vi "Main1.vi"(11 "Stage control":T2={"Up"=FALSE, "Left"=FALSE, "Right"=FALSE, "Down"=FALSE, "Z Down"=FALSE, "Z Up"=FALSE, "X Step Size(um)"=503.04, "Z step size (um)"=10.0, "Y Step Size(um)"=503.04, "Enable x-axis"=TRUE, "Enable y-axis"=TRUE, "Enable z-axis"=TRUE, "Same step size"=FALSE, "Global step size (um)"=10.0, "stop"=FALSE, "Destination"={"X Position"=-2.48414, "Y Position"=-11.8106, "Z Position"=5.53412}, "Move to destination"=FALSE}) -> (10 "Stage position":T1={"X Position"=-42.4711328125, "Y Position"=0.013554687499999999, "Z Position"=0.03555999999999933})   [LabVIEW 2020]
uses:
  typedefs/typedef_stage_control.ctl
  typedefs/typedef_stage_position.ctl
  typedefs/Laser_toggles__manual_typedef.ctl
  typedefs/typedef_voice_coil_function_generation.ctl
  typedefs/typedef_sawtooth_control.ctl
  typedefs/typedef_acquisition.ctl
  typedefs/typedef_laser_order_control.ctl
  <vilib>/DAQmx/write.llb/DAQmx Write (Analog DBL 1Chan 1Samp).vi
  Global stop DAQ.vi
  Global stop.vi
  Global Z-stack acquistion finished flag.vi
  Global DAQ started.vi
  Global destination achieved.vi
  Global stage boundaries.vi
  <vilib>/DAQmx/create/channels.llb/DAQmx Create Channel (AO-Voltage-Basic).vi
  <vilib>/DAQmx/miscellaneous.llb/DAQmx Fill In Error Info.vi
  Global Counter count.vi
panel:
  in  "error in":errorcluster
  in  "Tab Control":enum32{"Manual setup", "Acquisition", "Debug"}(tab)
  in  "Move Home":bool
  out "FirmwareVersion":string="3.03\r"
  out "Connected":bool
  in  "Laser Toggles":T3 {"Laser 642 nm power" min=0.0 max=5.0 scale=0.0..100.0; "Laser 595 nm power" min=0.0 max=5.0 scale=0.0..100.0; "Laser 560 nm power" min=0.0 max=5.0 scale=0.0..100.0; "Laser 488 nm power" min=0.0 max=5.0 scale=0.0..100.0}
  in  "Voice coil voltage slider":dbl(slide) min=-0.6 max=0.6 scale=-0.6..0.6
  in  "Voice coil \ncontrol mode":T4(ring)
  in  "Voice coil voltage output [V]":dbl min=-0.6 max=0.6 format="%#_3g"
  in  "Voice coil function generation":T5={"File to read"=path "C:/Users/Hannah/Downloads/calibration_0624_25msflyback.txt", "Image acquisition time (ms)"=1000.0, "Flyback time (ms)"=25.0}
  in  "Sawtooth generator":T6={"Amplitude [V]"=0.257, "Offset [V]"=-0.031, "Frequency (Hz)"=1.0} {"Frequency (Hz)" min=-50.0 max=50.0 step=0.00010000000000000003 format="%#_13g"; "Offset [V]" format="%.2p"; "Amplitude [V]" min=-0.7 max=0.7 format="%.2p"}
  in  "Calibrate home":bool
  in  "Abort acquisition":bool
  in  "Acquisition":T7={"Acquire"=FALSE, "Step size X and Y (um)"=598.88, "Number of tiles in X"=1.0, "Number of tiles in Y"=1.0, "Number of slices in Z"=1.0, "Step size Z (um)"=0.2, "Image acquisition time (ms)"=1000.0, "Flyback time (ms)"=25.0, "Moving time between tiles (ms)"=5000.0, "Total progress"=0, "Percentage overlap"=5.0, "Voice coil calibration file"=path "C:/Users/Hannah/Downloads/calibration1_fps_10000_samples_25ms_flyback", "Saved file location"=path "C:/Users/Hannah/Downloads/PositionLog7", "typedef_laser_order_control"={"Laser 560 nm order selection"=0, "Laser 595 nm order selection"=0, "Laser 642 nm order selection"=0, "Laser 488 nm order selection"=1, "Color Box"=60927, "Color Box 2"=12844800, "Color Box 3"=14132992, "Color Box 4"=16715008}, "Z-stack progress"=0} {"Z-stack progress" scale=0.0..100.0; "typedef_laser_order_control"."Laser 488 nm order selection" items=["Not active", "1", "2", "3", "4"]; "typedef_laser_order_control"."Laser 642 nm order selection" items=["Not active", "1", "2", "3", "4"]; "typedef_laser_order_control"."Laser 595 nm order selection" items=["Not active", "1", "2", "3", "4"]; "typedef_laser_order_control"."Laser 560 nm order selection" items=["Not active", "1", "2", "3", "4"]; "Percentage overlap" min=0.1 max=100.0; "Total progress" scale=0.0..100.0}
  out "Error out":errorcluster
  in  "DAQ Setup":enum16{"Test setup", "Microscope"}(ring)=enum."Microscope"
  in  "stop":bool
  out "Number of commands":i32=159
  out "waiting time (ms)":dbl
  out "output cluster":T9={"element"="acquire Zstack", "reference OUT"=refnum, "error OUT"={"status"=FALSE, "code"=0, "source"=""}}
  in  "additional delay":dbl=-97.0
  out "string array":string[](array[string])=["acquireXY", "WAIT2040", "MOVEX+1", "WAIT5000", "acquireXY", "WAIT2040", "MOVEX+1", "WAIT5000", "acquireXY", "WAIT2040", "MOVEX+1", "WAIT5000", "acquireXY", "WAIT2040", "MOVEY-1", "WAIT5000", "acquireXY", "WAIT2040", "MOVEX-1", "WAIT5000", "acquireXY", "WAIT2040", "MOVEX-1", "WAIT5000", "acquireXY", "WAIT2040", "MOVEX-1", "WAIT5000", "acquireXY", "WAIT2040", "MOVEY-1", "WAIT5000", "acquireXY", "WAIT2040", "MOVEX+1", "WAIT5000", "acquireXY", "WAIT2040", "MOVEX+1", "WAIT5000", "acquireXY", "WAIT2040", "MOVEX+1", "WAIT5000", "acquireXY", "WAIT2040", "MOVEY-1", "WAIT5000", "acquireXY", "WAIT2040", "MOVEX-1", "WAIT5000", "acquireXY", "WAIT2040", "MOVEX-1", "WAIT5000", "acquireXY", "WAIT2040", "MOVEX-1", "WAIT5000", "acquireXY", "WAIT2040", "MOVEY-1", "WAIT5000", "acquireXY", "WAIT2040", "MOVEX+1", "WAIT5000", "acquireXY", "WAIT2040", "MOVEX+1", "WAIT5000", "acquireXY", "WAIT2040", "MOVEX+1", "WAIT5000", "acquireXY", "WAIT2040", "MOVEY-1", "WAIT5000", "acquireXY", "WAIT2040", "MOVEX-1", "WAIT5000", "acquireXY", "WAIT2040", "MOVEX-1", "WAIT5000", "acquireXY", "WAIT2040", "MOVEX-1", "WAIT5000", "acquireXY", "WAIT2040", "MOVEY-1", "WAIT5000", "acquireXY", "WAIT2040", "MOVEX+1", "WAIT5000", "acquireXY", "WAIT2040", "MOVEX+1", "WAIT5000", "acquireXY", "WAIT2040", "MOVEX+1", "WAIT5000", "acquireXY", "WAIT2040", "MOVEY-1", "WAIT5000", "acquireXY", "WAIT2040", "MOVEX-1", "WAIT5000", "acquireXY", "WAIT2040", "MOVEX-1", "WAIT5000", "acquireXY", "WAIT2040", "MOVEX-1", "WAIT5000", "acquireXY", "WAIT2040", "MOVEY-1", "WAIT5000", "acquireXY", "WAIT2040", "MOVEX+1", "WAIT5000", "acquireXY", "WAIT2040", "MOVEX+1", "WAIT5000", "acquireXY", "WAIT2040", "MOVEX+1", "WAIT5000", "acquireXY", "WAIT2040", "MOVEY-1", "WAIT5000", "acquireXY", "WAIT2040", "MOVEX-1", "WAIT5000", "acquireXY", "WAIT2040", "MOVEX-1", "WAIT5000", "acquireXY", "WAIT2040", "MOVEX-1", "WAIT5000", "acquireXY", "WAIT2040", "end"]
  out "String":string="X+1 movement"
  out "Z-stack start position":T1
  in  "X-direction":enum16{"Up", "Down"}(ring)
  in  "Y-direction":enum16{"Left", "Right"}(ring)=enum."Right"
  out "Numeric 2":i32
  out "Boolean":bool
  out "Numeric 3":i32
  out "Numeric 4":i32
  out "Stage position OUT":T1
  out "Stage position OUT 2":T1
  in  "FOV (um)":dbl=630.4 format="%#_13g"
  out "current position in string array":i32=11
  in  "Camera trigger initial delay [ms]":dbl format="%.6f"
  out "Global Counter count":dbl
  out "Numeric":i32
  in  "SPIIPLUSCOM660Lib.IAsyncChannel":refnum<k7>
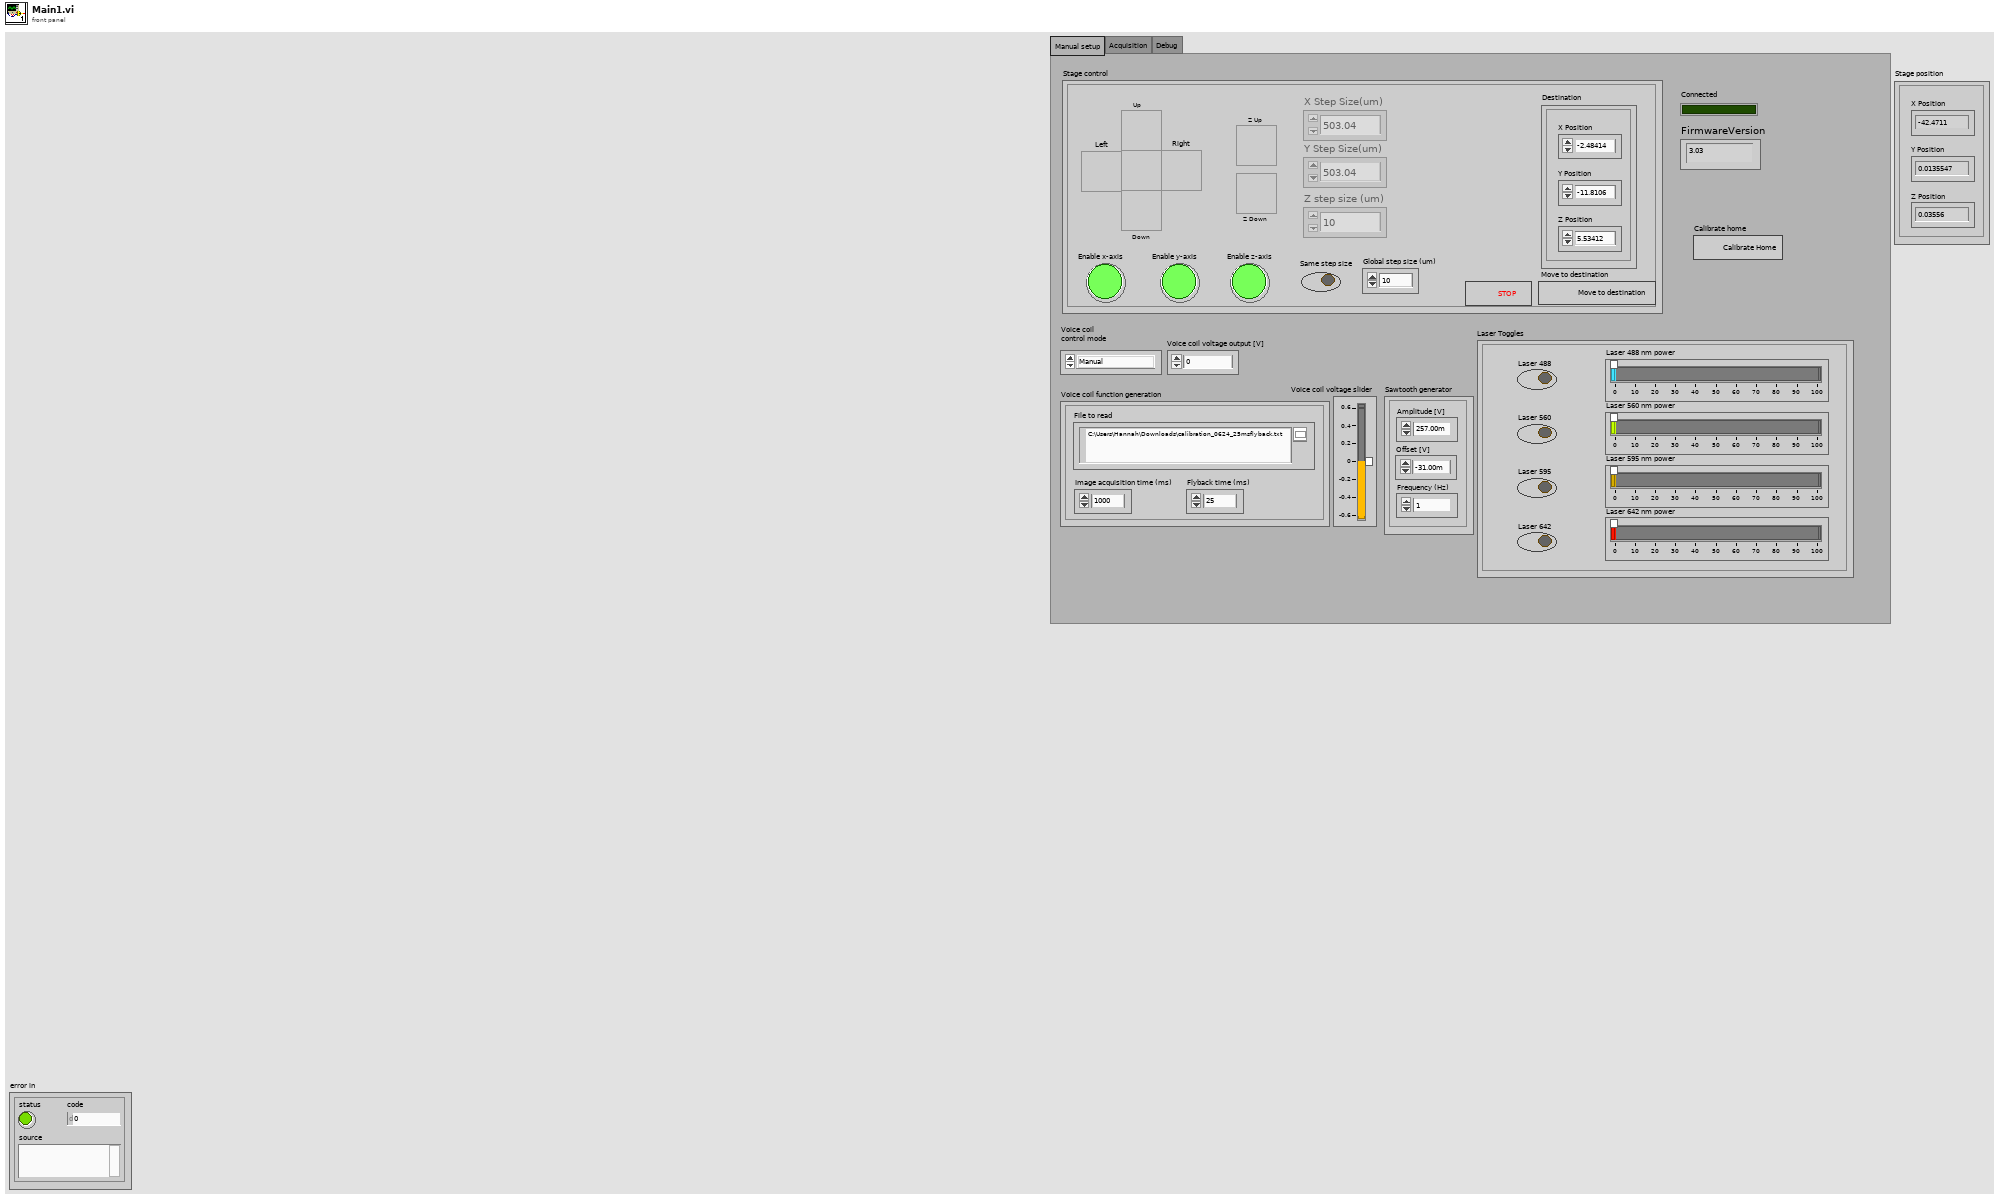
[diagram p1: front panel]
types:
  T1 = typedef "typedef_stage_position.ctl" = cluster{"X Position":dbl, "Y Position":dbl, "Z Position":dbl}
  T2 = typedef "typedef_stage_control.ctl" = cluster{"Up":bool, "Left":bool, "Right":bool, "Down":bool, "Z Down":bool, "Z Up":bool, "X Step Size(um)":dbl, "Z step size (um)":dbl, "Y Step Size(um)":dbl, "Enable x-axis":bool, "Enable y-axis":bool, "Enable z-axis":bool, "Same step size":bool, "Global step size (um)":dbl, "stop":bool, "Destination":T1, "Move to destination":bool}
  T3 = typedef "Laser_toggles__manual_typedef.ctl" = cluster{"Laser 488 nm power":dbl, "Laser 560 nm power":dbl, "Laser 595 nm power":dbl, "Laser 642 nm power":dbl, "Laser 560 ":bool, "Laser 595 ":bool, "Laser 642 ":bool, "Laser 488 ":bool}
  T4 = enum16{"Manual", "Saw tooth function", "From file"}
  T5 = typedef "typedef_voice_coil_function_generation.ctl" = cluster{"File to read":path, "Image acquisition time (ms)":dbl, "Flyback time (ms)":dbl}
  T6 = typedef "typedef_sawtooth_control.ctl" = cluster{"Amplitude [V]":dbl, "Offset [V]":dbl, "Frequency (Hz)":dbl}
  T7 = typedef "typedef_acquisition.ctl" = cluster{"Acquire":bool, "Step size X and Y (um)":dbl, "Number of tiles in X":dbl, "Number of tiles in Y":dbl, "Number of slices in Z":dbl, "Step size Z (um)":dbl, "Image acquisition time (ms)":dbl, "Flyback time (ms)":dbl, "Moving time between tiles (ms)":dbl, "Total progress":u8, "Percentage overlap":dbl, "Voice coil calibration file":path, "Saved file location":path, "typedef_laser_order_control":T8, "Z-stack progress":u8}
  T8 = typedef "typedef_laser_order_control.ctl" = cluster{"Laser 560 nm order selection":u16, "Laser 595 nm order selection":u16, "Laser 642 nm order selection":u16, "Laser 488 nm order selection":u16, "Color Box":u32, "Color Box 2":u32, "Color Box 3":u32, "Color Box 4":u32}
  T9 = cluster{"element":string, "reference OUT":refnum<k7>, "error OUT":errorcluster}
  T10 = enum16{"Initialize", "Verify connection", "Running", "Closing"}
  T11 = enum16{"Turn off X and Y", "Manually move stage 1", "Manually move stage 2", "Enable Home button", "Activate X and Y"}
  T12 = enum8{"Enabled", "Disabled", "Disabled and Grayed Out"}
  T13 = typedef "typedef_boundaries.ctl" = cluster{"X lower bound":dbl, "X upper bound":dbl, "Y lower bound":dbl, "Y upper bound ":dbl, "Z lower bound":dbl, "Z upper bound ":dbl}
  T14 = typedef "DAQ_channel_typedef.ctl" = cluster{"CO.Pulse.Term":tag, "Voice coil analog output":tag, "counter":tag, "CO.Pulse.Term 2":tag, "AOTF lines":tag, "counter 2":tag, "CO.Pulse.Term 3":tag, "counter 3":tag}
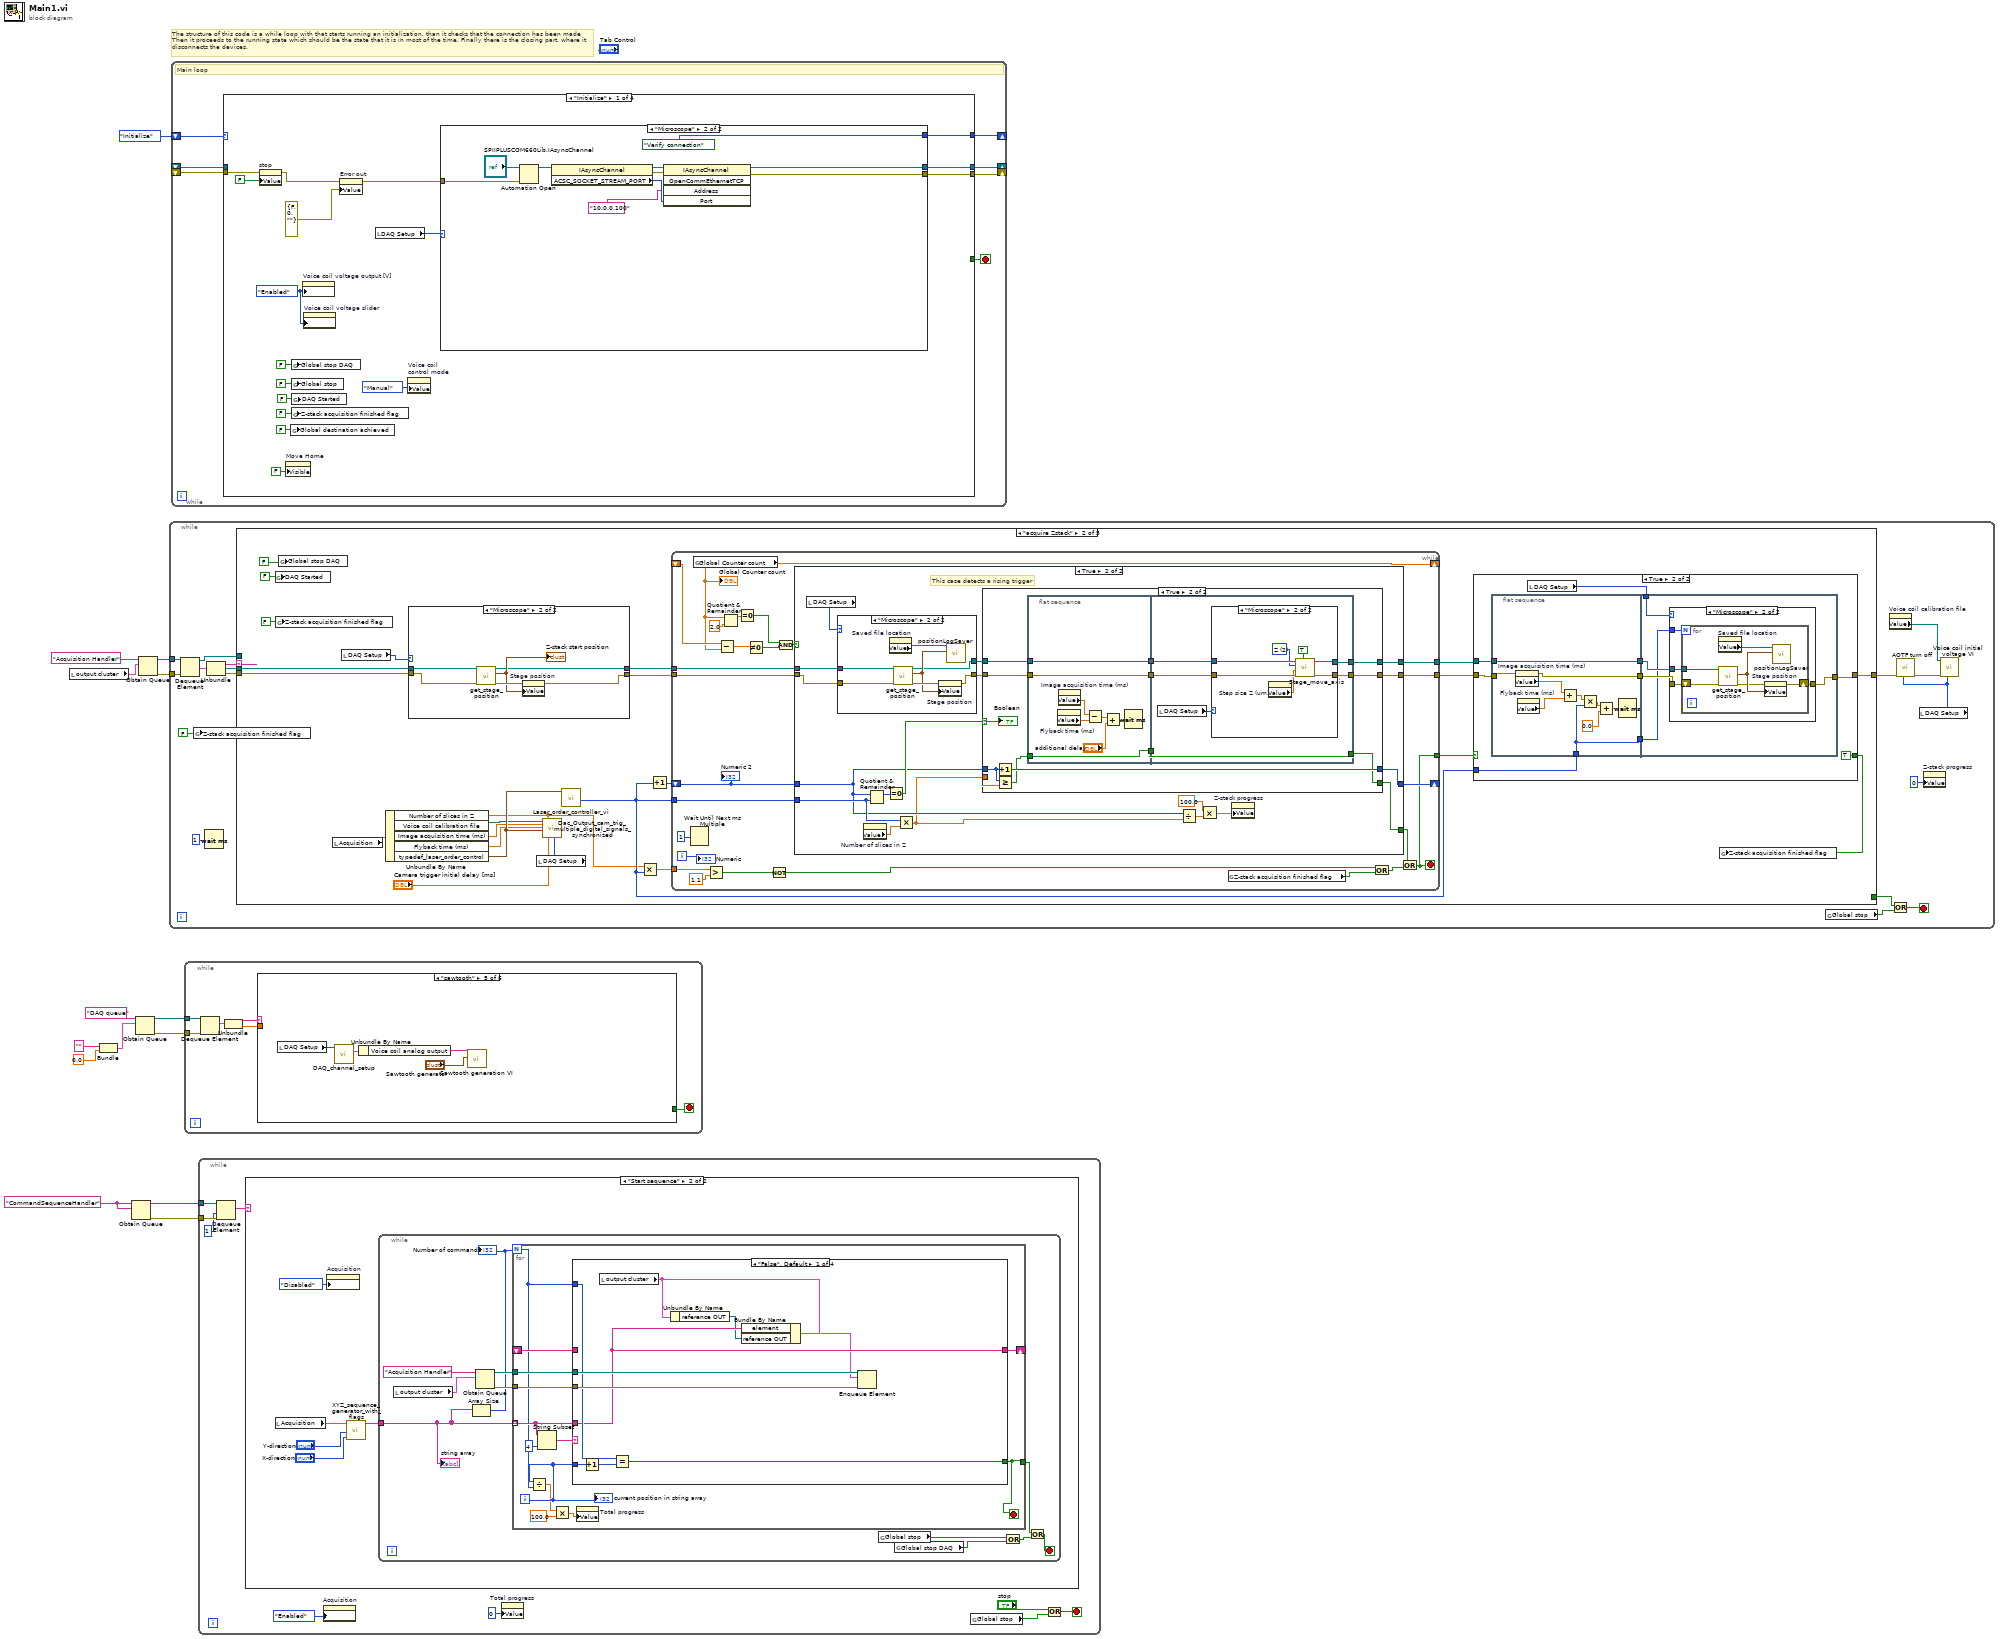
[diagram p0: block diagram]
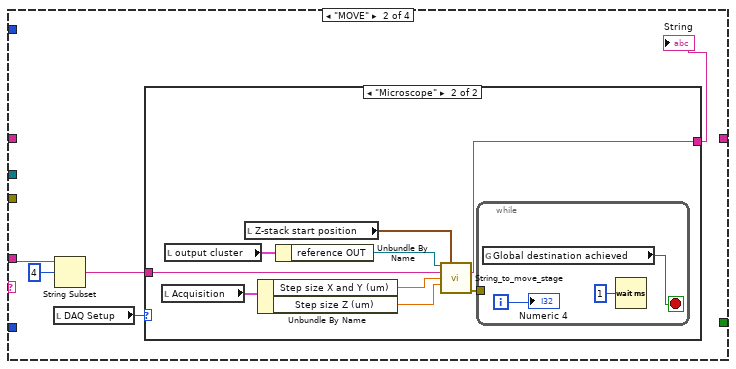
[diagram p3: hidden frame]
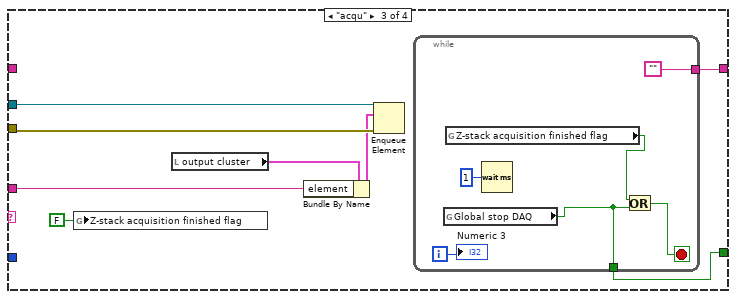
[diagram p5: hidden frame]
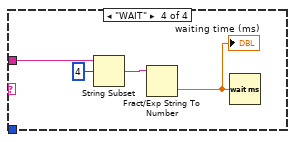
[diagram p6: hidden frame]
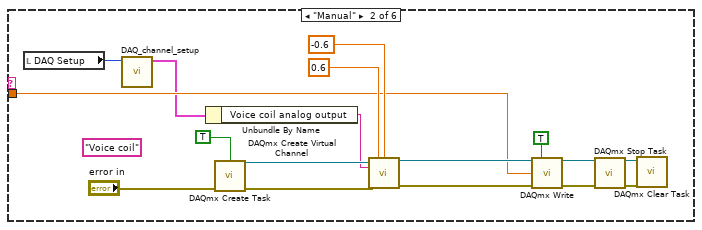
[diagram p8: hidden frame]
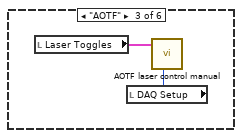
[diagram p9: hidden frame]
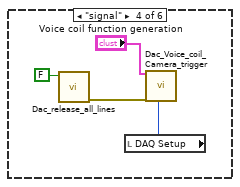
[diagram p10: hidden frame]
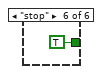
[diagram p11: hidden frame]
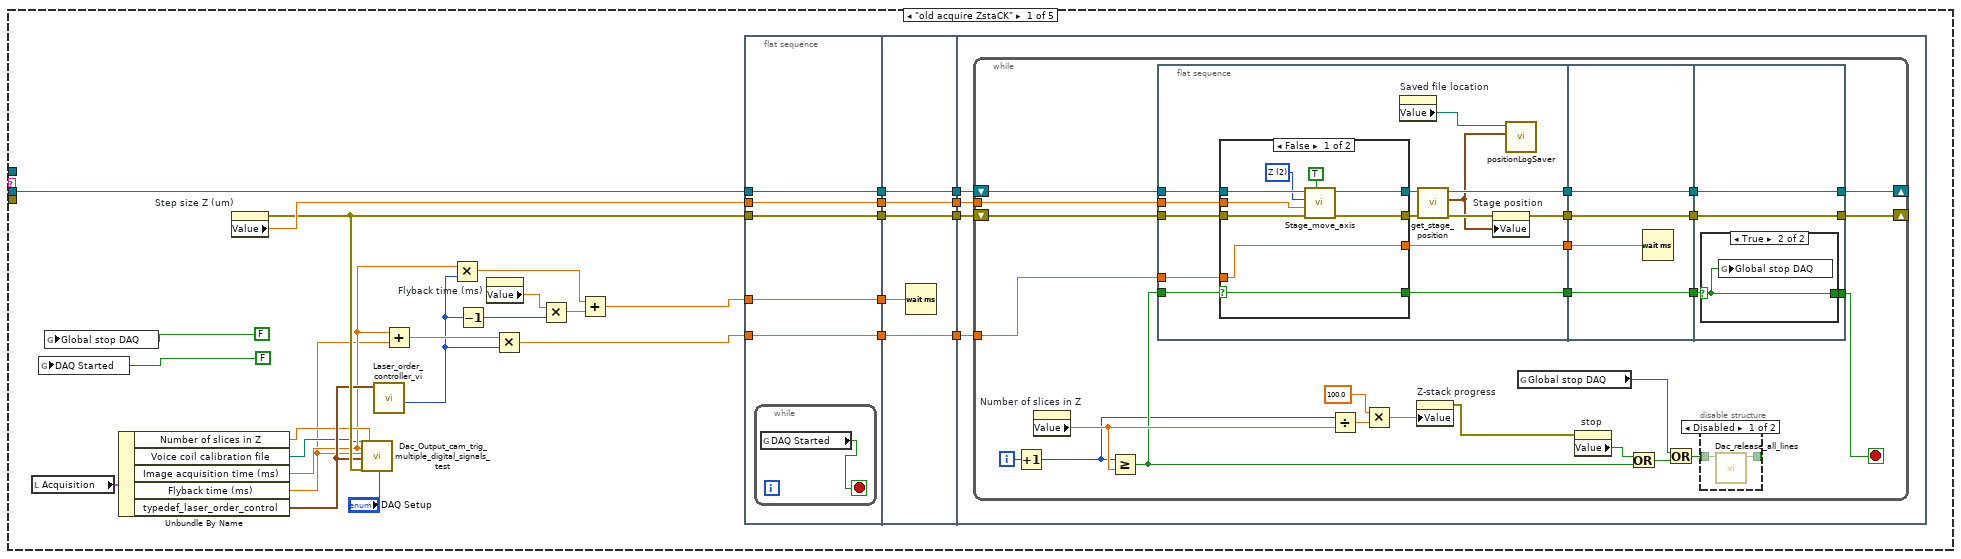
[diagram p12: hidden frame]
diagram:
  w2 = "CommandSequenceHandler" ("name (unnamed)")
  # "The structure of this code is a while loop with that starts running an initialization, than it checks that the connection has been made\nThen it proceeds to the running state which should be the state that it is in most of the time. Finally there is the closing part, where it\ndisconnects the devices."
  n1 = local read "output cluster"() -> (w1:T9)
  n2 = Bundle("", 0.0) -> (w10:cluster{string, dbl})  [unwired: 1 in]
  n3 = Obtain Queue(name (unnamed)=w2, element data type=w2) -> (queue out=w4:refnum<queue>, error out=w3:errorcluster)  [unwired: 3 in, 1 out]
  n4 = Obtain Queue(name (unnamed)="DAQ queue", element data type=w10) -> (queue out=w8:refnum<queue>, error out=w7:errorcluster)  [unwired: 3 in, 1 out]
  n5 = Obtain Queue(name (unnamed)="Acquisition Handler", element data type=w1) -> (queue out=w12:refnum<queue>, error out=w11:errorcluster)  [unwired: 3 in, 1 out]
  n6 = while {
    tunnel: w12 -> [w31]
    tunnel: w11 -> [w30]
    stop <- w19 stop-if-true
    n7 = Dequeue Element(queue=w31, error in (no error)=w30) -> (queue out=w25:refnum<queue>, element=w29:T9)  [unwired: 1 in, 2 out]
    n8 = global write "Global Z-stack acquistion finished flag.vi" "Z-stack acquisition finished flag"(FALSE ("Z-stack acquisition finished flag")) -> ()
    n9 = Wait (ms)(milliseconds to wait=u32 1) -> ()  [unwired: 1 out]
    n10 = Unbundle(w29) -> ("element"=w28:string, "reference OUT"=w27:refnum<k7>, "error OUT"=w26:errorcluster)
    n11 = case shown="\"acquire Zstack\"" w28 {
      tunnel: w27 -> [w60 w162 _ _ _]
      tunnel: w26 -> [_ w161 _ _ _]
      tunnel: [_ _ _ _ TRUE] -> w18
      tunnel: w25 -> [_ _ _ _ _]
      tunnel: [_ w152 _ _ _] -> w15
      frame "old acquire ZstaCK" {
        n12 = local read "Acquisition"() -> (w36:T7)
        n13 = global write "Global DAQ started.vi" "DAQ Started"(FALSE ("DAQ Started")) -> ()
        n14 = global write "Global stop DAQ.vi" "Global stop DAQ"(FALSE ("Global stop DAQ")) -> ()
        n15 = Unbundle By Name(w36) -> ("Number of slices in Z"=w35:dbl, "Voice coil calibration file"=w33:path, "Image acquisition time (ms)"=w34:dbl, "Flyback time (ms)"=w32:dbl, "typedef_laser_order_control"=w37:T8)
        n16 = property on="Step size Z (um)" class="DigNum (strict)"() -> (error out=w58:errorcluster, "Value"=w59:dbl)  [unwired: 2 in, 1 out]
        n17 = call "Dac_Output_cam_trig_multiple_digital_signals_test.vi"("File to read"=w33, "Image acquisition time (ms)"=w34, "Delay between frames"=w32, "typedef_laser_order_control"=w37, "error in"=w58, "Number of slices"=w35, "Setup"="DAQ Setup") -> ()  [unwired: 12 in, 1 out]
        n18 = call "Laser_order_controller_vi.vi"("typedef_laser_order_control"=w37) -> ("Active lasers"=w39:i16)  [unwired: 8 in, 2 out]
        n19 = Add(x=w34, y=w32) -> (x+y=w57:dbl)
        n20 = Multiply(x=w34, y=w39) -> (x*y=w38:dbl)
        n21 = Decrement(x=w39) -> (x-1=w54:i16)
        n22 = property on="Flyback time (ms)" class="DigNum (strict)"() -> ("Value"=w53:dbl)  [unwired: 2 in, 2 out]
        n23 = Multiply(x=w57, y=w39) -> (x*y=w51:dbl)
        n24 = Multiply(x=w53, y=w54) -> (x*y=w52:dbl)
        n25 = Add(x=w38, y=w52) -> (x+y=w46:dbl)
        n26 = flat-sequence {
          tunnel: w46 -> [w61]
          tunnel: w51 -> [w62]
          tunnel: w58 -> [w63]
          tunnel: w59 -> [w64]
          tunnel: w60 -> [w65]
          tunnel: [w65] -> w45
          tunnel: [w64] -> w44
          tunnel: [w63] -> w43
          tunnel: [w62] -> w42
          tunnel: [w61] -> w41
          tunnel: [w71] -> w50
          tunnel: [w70] -> w49
          tunnel: [w69] -> w48
          tunnel: [w68] -> w47
          tunnel: w45 -> [w71]
          tunnel: w44 -> [w70]
          tunnel: w43 -> [w69]
          tunnel: w42 -> [w68]
          tunnel: w41 -> [w67]
          tunnel: w50 -> [w75]
          tunnel: w49 -> [w74]
          tunnel: w48 -> [w73]
          tunnel: w47 -> [w72]
          frame #0 {
            n27 = while {
              stop <- w66 stop-if-true
              n28 = global read "Global DAQ started.vi" "DAQ Started"() -> (w66:bool)
            }
          }
          frame #1 {
            n29 = Wait (ms)(milliseconds to wait=w67) -> ()  [unwired: 1 out]
          }
          frame #2 {
            n30 = while {
              shift-right: [w100] -> _
              shift-left: w75 -> [w101]
              shift-right: [w84] -> _
              shift-left: w73 -> [w90]
              tunnel: w74 -> [w96]
              tunnel: w72 -> [w88]
              i -> [w82]
              stop <- w77 stop-if-true
              n31 = Increment(x=w82) -> (x+1=w76:i32)
              n32 = property on="Number of slices in Z" class="DigNum (strict)"() -> ("Value"=w94:dbl)  [unwired: 2 in, 2 out]
              n33 = Greater Or Equal?(x=w76, y=w94) -> (x >= y?=w83:bool)
              n34 = flat-sequence {
                tunnel: w101 -> [w118]
                tunnel: w96 -> [w115]
                tunnel: [w117] -> w93
                tunnel: [w116] -> w92
                tunnel: w90 -> [w111]
                tunnel: w83 -> [w110]
                tunnel: w88 -> [w109]
                tunnel: [w108] -> w89
                tunnel: [w106] -> w78
                tunnel: w93 -> [w135]
                tunnel: w92 -> [w134]
                tunnel: w89 -> [w132]
                tunnel: [w135] -> w81
                tunnel: [w134] -> w80
                tunnel: [w133] -> w79
                tunnel: w78 -> [w133]
                tunnel: [w138] -> w84
                tunnel: [w139] -> w100
                tunnel: w81 -> [w139]
                tunnel: w80 -> [w138]
                tunnel: w79 -> [w137]
                tunnel: [w136] -> w77
                frame #0 {
                  n35 = case shown="False" w110 {
                    selector: w110 -> [w120 w129]
                    tunnel: w118 -> [w127 w131]
                    tunnel: w115 -> [w126 _]
                    tunnel: [w123 w131] -> w114
                    tunnel: [w122 w130] -> w113
                    tunnel: w111 -> [w121 w130]
                    tunnel: w109 -> [w119 w128]
                    tunnel: [w119 w128] -> w108
                    tunnel: [w120 w129] -> w106
                    frame False {
                      w125 = u16 2 items=["X", "Y", "Z"] ("Axes Select")
                      n36 = call "Stage_move_axis.vi"("Direction true means positive increment"=TRUE, "error in (no error)"=w121, "Distance micrometer"=w126, "Axes Select"=w125, "reference IN"=w127) -> ("error OUT"=w122:errorcluster, "reference OUT"=w123:refnum<k7>)  [unwired: 5 in]
                    }
                    frame True {
                      # "Last acquisition should not wait"
                    }
                  }
                  n37 = property on="Saved file location" class="Path"() -> ("Value"=w105:path)  [unwired: 2 in, 2 out]
                  n38 = call "get_stage_position.vi"("error IN"=w113, "reference IN"=w114) -> ("error OUT"=w112:errorcluster, "Stage position OUT"=w107:T1, "reference OUT"=w117:refnum<k7>)  [unwired: 7 in]
                  n39 = property on="Stage position" class="Clust (strict)"(error in=w112, "Value"=w107) -> (error out=w116:errorcluster)  [unwired: 1 in, 1 out]
                  n40 = call "positionLogSaver.vi"("Stage position"=w107, "file path (use dialog)"=w105) -> ()  [unwired: 10 in]
                }
                frame #1 {
                  n41 = Wait (ms)(milliseconds to wait=w132) -> ()  [unwired: 1 out]
                }
                frame #2 {
                  n42 = case shown="True" w137 {
                    selector: w137 -> [w140 w141]
                    tunnel: [w140 w141] -> w136
                    frame False {
                    }
                    frame True {
                      n43 = global write "Global stop DAQ.vi" "Global stop DAQ"(w141) -> ()
                    }
                  }
                }
              }
              n44 = Divide(x=w76, y=w94) -> (x/y=w98:dbl)
              n45 = Multiply(x=100.0 ("y"), y=w98) -> (x*y=w95:dbl)
              n46 = property on="Z-stack progress" class="Slide (strict)"("Value"=w95) -> (error out=w91:errorcluster)  [unwired: 2 in, 1 out]
              n47 = global read "Global stop DAQ.vi" "Global stop DAQ"() -> (w86:bool)
              n48 = property on="stop" class="Bool (strict)"(error in=w91) -> ("Value"=w99:bool)  [unwired: 1 in, 2 out]
              n49 = Or(x=w99, y=w83) -> (x .or. y?=w87:bool)
              n50 = Or(x=w86, y=w87) -> (x .or. y?=w85:bool)
              n51 = disable-structure shown="Disabled" {
                disable-tunnel: w85 -> [w103 w104]
                disable-tunnel: [w102 w104] -> _
                frame Disabled {
                  n52 = call "Dac_release_all_lines.vi"("Release all DAQ lines"=w103) -> ("Finished"=w102:bool)  [unwired: 9 in, 1 out]
                }
                frame Enabled {
                }
              }
            }
          }
        }
      }
      frame "acquire Zstack" {
        n53 = global write "Global DAQ started.vi" "DAQ Started"(FALSE ("DAQ Started")) -> ()
        n54 = global write "Global Z-stack acquistion finished flag.vi" "Z-stack acquisition finished flag"(FALSE ("Z-stack acquisition finished flag")) -> ()
        n55 = global write "Global stop DAQ.vi" "Global stop DAQ"(FALSE ("Global stop DAQ")) -> ()
        n56 = local read "Acquisition"() -> (w148:T7)
        n57 = local read "DAQ Setup"() -> (w157:enum16{"Test setup", "Microscope"})
        n58 = Unbundle By Name(w148) -> ("Number of slices in Z"=w143:dbl, "Voice coil calibration file"=w146:path, "Image acquisition time (ms)"=w144:dbl, "Flyback time (ms)"=w145:dbl, "typedef_laser_order_control"=w147:T8)
        n59 = case shown="\"Microscope\"" w157 {
          tunnel: w162 -> [w204 w208]
          tunnel: w161 -> [w203 w207]
          tunnel: [w203 w206] -> w160
          tunnel: [w204 w205] -> w159
          frame "Test setup", Default {
          }
          frame "Microscope" {
            n60 = call "get_stage_position.vi"("error IN"=w207, "reference IN"=w208) -> ("error OUT"=w210:errorcluster, "Stage position OUT"=w209:T1, "reference OUT"=w205:refnum<k7>)  [unwired: 7 in]
            "Z-stack start position" <- w209
            n61 = property on="Stage position" class="Clust (strict)"(error in=w210, "Value"=w209) -> (error out=w206:errorcluster)  [unwired: 1 in, 1 out]
          }
        }
        n62 = local read "DAQ Setup"() -> (w163:enum16{"Test setup", "Microscope"})
        n63 = call "Dac_Output_cam_trig_multiple_digital_signals_synchronized.vi"("File to read"=w146, "Image acquisition time (ms)"=w144, "Delay between frames (ms)"=w145, "typedef_laser_order_control"=w147, "Number of slices"=w143, "Camera trigger initial delay [ms]"="Camera trigger initial delay [ms]", "Setup"=w163) -> ()  [unwired: 12 in, 1 out]
        n64 = call "Laser_order_controller_vi.vi"("typedef_laser_order_control"=w147) -> ("Active lasers"=w149:i16)  [unwired: 8 in, 2 out]
        n65 = Multiply(x=w143, y=w149) -> (x*y=w155:dbl)
        n66 = Increment(x=w149) -> (x+1=w150:i16)
        n67 = while {
          shift-right: [w226] -> _
          shift-left: _ -> [w228]
          tunnel: w159 -> [w234]
          tunnel: w160 -> [w233]
          shift-right: [w229] -> _
          shift-left: w150 -> [w230]
          tunnel: w149 -> [w224]
          tunnel: [w223] -> w154
          tunnel: w155 -> [w222]
          tunnel: [w215] -> w156
          tunnel: [w214] -> w153
          i -> [w231]
          stop <- w215 stop-if-true
          n68 = Wait Until Next ms Multiple(millisecond multiple=u32 1) -> ()  [unwired: 1 out]
          n69 = global read "Global Counter count.vi" "Global Counter count"() -> (w226:dbl)
          "Global Counter count" <- w226
          n70 = Greater?(x=w222, y=1.1) -> (0:w217:bool)
          n71 = Subtract(x=w228, y=w226) -> (x-y=w235:dbl)
          n72 = Quotient & Remainder(x=w226, y=2.0) -> (x-y*floor(x/y)=w225:dbl)  [unwired: 1 out]
          n73 = Equal To 0?(x=w225) -> (x = 0?=w219:bool)
          n74 = Not Equal To 0?(x=w235) -> (x != 0?=w218:bool)
          n75 = Not(x=w217) -> (.not. x?=w212:bool)
          n76 = And(x=w219, y=w218) -> (x .and. y?=w220:bool)
          n77 = case shown="True" w220 {
            tunnel: w234 -> [w236 w242]
            tunnel: w233 -> [w237 w243]
            tunnel: w230 -> [w238 w247]
            tunnel: [w238 w246] -> w229
            tunnel: w224 -> [_ w250]
            tunnel: [_ w244] -> w216
            tunnel: [w237 w249] -> w223
            tunnel: [w236 w248] -> w214
            frame False {
            }
            frame True {
              # "This case detects a rising trigger"
              n78 = local read "DAQ Setup"() -> (w239:enum16{"Test setup", "Microscope"})
              n79 = case shown="\"Microscope\"" w239 {
                tunnel: w243 -> [w257 w262]
                tunnel: w242 -> [w258 w261]
                tunnel: [w257 w260] -> w241
                tunnel: [w258 w259] -> w240
                frame "Test setup", Default {
                }
                frame "Microscope" {
                  n80 = property on="Saved file location" class="Path"() -> ("Value"=w265:path)  [unwired: 2 in, 2 out]
                  n81 = call "get_stage_position.vi"("error IN"=w262, "reference IN"=w261) -> ("error OUT"=w264:errorcluster, "Stage position OUT"=w263:T1, "reference OUT"=w259:refnum<k7>)  [unwired: 7 in]
                  n82 = property on="Stage position" class="Clust (strict)"(error in=w264, "Value"=w263) -> (error out=w260:errorcluster)  [unwired: 1 in, 1 out]
                  n83 = call "positionLogSaver.vi"("Stage position"=w263, "file path (use dialog)"=w265) -> ()  [unwired: 10 in]
                }
              }
              n84 = property on="Number of slices in Z" class="DigNum (strict)"() -> ("Value"=w251:dbl)  [unwired: 2 in, 2 out]
              n85 = Quotient & Remainder(x=w247, y=w250) -> (x-y*floor(x/y)=w253:i16)  [unwired: 1 out]
              n86 = Equal To 0?(x=w253) -> (x = 0?=w252:bool)
              n87 = Multiply(x=w250, y=w251) -> (x*y=w245:dbl)
              n88 = case shown="True" w252 {
                selector: w252 -> [w270 w281]
                tunnel: [w271 w284] -> w249
                tunnel: w240 -> [w269 w283]
                tunnel: w241 -> [w271 w282]
                tunnel: [w269 w278] -> w248
                tunnel: w247 -> [w267 w276]
                tunnel: [w268 w277] -> w246
                tunnel: w245 -> [_ w275]
                tunnel: [FALSE w272] -> w244
                frame False {
                  n89 = local write "Boolean"(w270) -> ()
                  n90 = Increment(x=w267) -> (x+1=w268:i16)
                }
                frame True {
                  n91 = Increment(x=w276) -> (x+1=w277:i16)
                  n92 = Greater Or Equal?(x=w276, y=w275) -> (x >= y?=w274:bool)
                  n93 = flat-sequence {
                    tunnel: w282 -> [w291]
                    tunnel: w283 -> [w292]
                    tunnel: [w292] -> w280
                    tunnel: [w291] -> w279
                    tunnel: w274 -> [w285]
                    tunnel: [w285] -> w273
                    tunnel: [w298] -> w284
                    tunnel: w280 -> [w297]
                    tunnel: w279 -> [w296]
                    tunnel: [w294] -> w278
                    tunnel: [w293] -> w272
                    tunnel: w273 -> [w293]
                    frame #0 {
                      n94 = property on="Flyback time (ms)" class="DigNum (strict)"() -> ("Value"=w289:dbl)  [unwired: 2 in, 2 out]
                      n95 = property on="Image acquisition time (ms)" class="DigNum (strict)"() -> ("Value"=w290:dbl)  [unwired: 2 in, 2 out]
                      n96 = Subtract(x=w290, y=w289) -> (x-y=w287:dbl)
                      n97 = Add(x=w287, y="additional delay") -> (x+y=w288:dbl)
                      n98 = Wait (ms)(milliseconds to wait=w288) -> ()  [unwired: 1 out]
                    }
                    frame #1 {
                      n99 = local read "DAQ Setup"() -> (w295:enum16{"Test setup", "Microscope"})
                      n100 = case shown="\"Microscope\"" w295 {
                        tunnel: [w300 w301] -> w298
                        tunnel: w297 -> [w299 w307]
                        tunnel: w296 -> [w300 w306]
                        tunnel: [w299 w302] -> w294
                        frame "Test setup", Default {
                        }
                        frame "Microscope" {
                          w305 = u16 2 items=["X", "Y", "Z"] ("Axes Select")
                          n101 = property on="Step size Z (um)" class="DigNum (strict)"() -> ("Value"=w303:dbl)  [unwired: 2 in, 2 out]
                          n102 = call "Stage_move_axis.vi"("Direction true means positive increment"=TRUE, "error in (no error)"=w306, "Distance micrometer"=w303, "Axes Select"=w305, "reference IN"=w307) -> ("error OUT"=w301:errorcluster, "reference OUT"=w302:refnum<k7>)  [unwired: 5 in]
                        }
                      }
                    }
                  }
                  "Boolean" <- w281
                }
              }
              n103 = Divide(x=w247, y=w245) -> (x/y=w256:dbl)
              n104 = Multiply(x=100.0 ("y"), y=w256) -> (x*y=w254:dbl)
              n105 = property on="Z-stack progress" class="Slide (strict)"("Value"=w254) -> ()  [unwired: 2 in, 2 out]
            }
          }
          n106 = global read "Global Z-stack acquistion finished flag.vi" "Z-stack acquisition finished flag"() -> (w211:bool)
          n107 = Or(x=w212, y=w211) -> (x .or. y?=w213:bool)
          n108 = Or(x=w216, y=w213) -> (x .or. y?=w215:bool)
          "Numeric" <- w231
          "Numeric 2" <- w230
        }
        n109 = case shown="True" w156 {
          selector: w156 -> [w167 _]
          tunnel: [w167 TRUE] -> w151
          tunnel: w149 -> [_ w172]
          tunnel: w154 -> [w166 w175]
          tunnel: w153 -> [_ w169]
          tunnel: [w166 w171] -> w152
          frame False {
          }
          frame True {
            n110 = flat-sequence {
              tunnel: w175 -> [w184]
              tunnel: w172 -> [w177]
              tunnel: [w183] -> w174
              tunnel: [w178] -> w170
              tunnel: w169 -> [w178]
              tunnel: [w177] -> w168
              tunnel: w174 -> [w190]
              tunnel: w173 -> [w191]
              tunnel: [w189] -> w171
              tunnel: w170 -> [w188]
              tunnel: w168 -> [w187]
              frame #0 {
                n111 = property on="Image acquisition time (ms)" class="DigNum (strict)"(error in=w184) -> (error out=w183:errorcluster, "Value"=w186:dbl)  [unwired: 1 in, 1 out]
                n112 = property on="Flyback time (ms)" class="DigNum (strict)"() -> ("Value"=w180:dbl)  [unwired: 2 in, 2 out]
                n113 = Add(x=w186, y=w180) -> (x+y=w185:dbl)
                n114 = Multiply(x=w185, y=w177) -> (x*y=w182:dbl)
                n115 = Add(x=w182, y=0.0) -> (x+y=w181:dbl)
                n116 = Wait (ms)(milliseconds to wait=w181) -> ()  [unwired: 1 out]
              }
              frame #1 {
                n117 = case shown="\"Microscope\"" w191 {
                  tunnel: [w192 w196] -> w189
                  tunnel: w190 -> [w192 w195]
                  tunnel: w188 -> [_ w194]
                  tunnel: w187 -> [_ w193]
                  frame "Test setup", Default {
                  }
                  frame "Microscope" {
                    n118 = for {
                      N: w193 -> [_]
                      shift-right: [w200] -> w196
                      shift-left: w195 -> [w199]
                      tunnel: w194 -> [w197]
                      n119 = property on="Saved file location" class="Path"() -> ("Value"=w198:path)  [unwired: 2 in, 2 out]
                      n120 = call "get_stage_position.vi"("error IN"=w199, "reference IN"=w197) -> ("error OUT"=w201:errorcluster, "Stage position OUT"=w202:T1)  [unwired: 7 in, 1 out]
                      n121 = property on="Stage position" class="Clust (strict)"(error in=w201, "Value"=w202) -> (error out=w200:errorcluster)  [unwired: 1 in, 1 out]
                      n122 = call "positionLogSaver.vi"("Stage position"=w202, "file path (use dialog)"=w198) -> ()  [unwired: 10 in]
                    }
                  }
                }
              }
            }
            n123 = local read "DAQ Setup"() -> (w173:enum16{"Test setup", "Microscope"})
          }
        }
        n124 = global write "Global Z-stack acquistion finished flag.vi" "Z-stack acquisition finished flag"(w151) -> ()
      }
      frame "acquireXY" {
        n125 = flat-sequence {
          tunnel: [w315] -> w311
          tunnel: [w320] -> w309
          tunnel: w311 -> [w323]
          tunnel: [w323] -> w310
          tunnel: w309 -> [w322]
          tunnel: [w322] -> w308
          tunnel: w310 -> [w325]
          tunnel: w308 -> [w324]
          frame #0 {
            n126 = global write "Global stop DAQ.vi" "Global stop DAQ"(FALSE ("Global stop DAQ")) -> ()
          }
          frame #1 {
            n127 = property on="Saved file location" class="Path"() -> ("Value"=w313:path)  [unwired: 2 in, 2 out]
            n128 = property on="Stage position" class="Clust (strict)"() -> ("Value"=w314:T1)  [unwired: 2 in, 2 out]
            n129 = call "positionLogSaver.vi"("Stage position"=w314, "file path (use dialog)"=w313) -> ()  [unwired: 10 in]
          }
          frame #2 {
            n130 = local read "Acquisition"() -> (w319:T7)
            n131 = Unbundle By Name(w319) -> ("Voice coil calibration file"=w315:path, "Image acquisition time (ms)"=w316:dbl, "Flyback time (ms)"=w317:dbl, "typedef_laser_order_control"=w318:T8)
            n132 = local read "DAQ Setup"() -> (w320:enum16{"Test setup", "Microscope"})
            n133 = call "Dac_Output_cam_trig_multiple_digital_signals.vi"("File to read"=w315, "Image acquisition time (ms)"=w316, "Delay between frames"=w317, "typedef_laser_order_control"=w318, "Setup"=w320) -> ()  [unwired: 14 in, 1 out]
          }
          frame #3 {
            n134 = Wait (ms)(milliseconds to wait=u32 0) -> ()  [unwired: 1 out]
          }
          frame #4 {
            n135 = call "Voice coil initial voltage VI.vi"("File Path"=w325, "DAQ Setup"=w324) -> ()  [unwired: 9 in]
          }
          frame #5 {
            n136 = global write "Global stop DAQ.vi" "Global stop DAQ"(TRUE ("Global stop DAQ")) -> ()
          }
          frame #6 {
            n137 = global write "Global stop DAQ.vi" "Global stop DAQ"(FALSE ("Global stop DAQ")) -> ()
          }
        }
      }
      frame Default {
      }
      frame "stop" {
      }
    }
    n138 = global read "Global stop.vi" "Global stop"() -> (w17:bool)
    n139 = property on="Voice coil calibration file" class="Path"() -> ("Value"=w16:path)  [unwired: 2 in, 2 out]
    n140 = Or(x=w18, y=w17) -> (x .or. y?=w19:bool)
    n141 = local read "DAQ Setup"() -> (w22:enum16{"Test setup", "Microscope"})
    n142 = call "AOTF turn off.vi"("error in"=w15, "DAQ Setup"=w22) -> ("error out"=w21:errorcluster)  [unwired: 8 in]
    n143 = property on="Z-stack progress" class="Slide (strict)"("Value"=u8 0) -> ()  [unwired: 2 in, 2 out]
    n144 = call "Voice coil initial voltage VI.vi"("File Path"=w16, "error in"=w21, "DAQ Setup"=w22) -> ()  [unwired: 8 in]
  }
  n145 = while {
    shift-right: [w331] -> _
    shift-left: T10."Initialize" -> [w334]
    shift-right: [w333] -> _
    shift-left: _ -> [w330]
    shift-right: [w332] -> _
    shift-left: _ -> [w329]
    stop <- w335 stop-if-true
    # "Main loop"
    n146 = case shown="\"Initialize\"" w334 {
      tunnel: [_ _ _ TRUE ("NewVal")] -> w335
      tunnel: [w352 w369 w405 _] -> w333
      tunnel: [w351 w367 w404 _] -> w332
      tunnel: [w350 w368 w411 _] -> w331
      tunnel: w330 -> [_ w373 w408 w760]
      tunnel: w329 -> [w348 w372 w407 w759]
      frame "Initialize" {
        w344 = T12."Enabled" ("Disabled")
        n147 = property on="stop" class="Bool (strict)"(error in=w348, "Value"=FALSE) -> (error out=w346:errorcluster)  [unwired: 1 in, 1 out]
        n148 = property on="Move Home" class="Bool (strict)"("Visible"=FALSE) -> ()  [unwired: 2 in, 2 out]
        n149 = global write "Global destination achieved.vi" "Global destination achieved"(FALSE ("Global destination achieved")) -> ()
        n150 = global write "Global stop DAQ.vi" "Global stop DAQ"(FALSE ("Global stop DAQ")) -> ()
        n151 = global write "Global stop.vi" "Global stop"(FALSE ("Global stop")) -> ()
        n152 = global write "Global Z-stack acquistion finished flag.vi" "Z-stack acquisition finished flag"(FALSE ("Z-stack acquisition finished flag")) -> ()
        n153 = global write "Global DAQ started.vi" "DAQ Started"(FALSE ("DAQ Started")) -> ()
        n154 = property on="Voice coil voltage output [V]" class="DigNum (strict)"("DisabledEnum"=w344) -> ()  [unwired: 2 in, 2 out]
        n155 = property on="Voice coil voltage slider" class="Slide (strict)"("DisabledEnum"=w344) -> ()  [unwired: 2 in, 2 out]
        n156 = property on="Error out" class="Clust (strict)"(error in=w346, "Value"=errorcluster {"status"=FALSE, "code"=0, "source"=""} ("Error out")) -> (error out=w345:errorcluster)  [unwired: 1 in, 1 out]
        n157 = local read "DAQ Setup"() -> (w341:enum16{"Test setup", "Microscope"})
        n158 = property on="Voice coil \ncontrol mode" class="Enum (strict)"("Value"=T4."Manual" ("Voice coil \ncontrol mode")) -> ()  [unwired: 2 in, 2 out]
        n159 = case shown="\"Microscope\"" w341 {
          tunnel: [_ w359] -> w352
          tunnel: [_ w358] -> w351
          tunnel: [T10."Running" T10."Verify connection"] -> w350
          tunnel: w345 -> [_ w356]
          frame "Test setup", Default {
            w353 = path "C:/Users/lpk27/Documents/ASLM/Image data/calibration_FPS_1_Flyback_25_ms.txt" ("Voice coil calibration file")
            n160 = property on="File to read" class="Path"("Value"=w353) -> ()  [unwired: 2 in, 2 out]
            n161 = property on="Voice coil calibration file" class="Path"("Value"=w353) -> ()  [unwired: 2 in, 2 out]
            n162 = property on="Saved file location" class="Path"("Value"=path "C:/Users/lpk27/Downloads/positionLog" ("Position log file location")) -> ()  [unwired: 2 in, 2 out]
          }
          frame "Microscope" {
            n163 = Automation Open(error in (no error)=w356, Automation Refnum="SPIIPLUSCOM660Lib.IAsyncChannel") -> (Automation Refnum=w365:refnum<k7>)  [unwired: 2 in, 1 out]
            n164 = property class="IAsyncChannel"(reference=w365) -> (reference out=w364:refnum<k7>, error out=w360:errorcluster, "ACSC_SOCKET_STREAM_PORT"=w362:i32)  [unwired: 1 in]
            n165 = invoke class="IAsyncChannel" method="OpenCommEthernetTCP"(reference=w364, error in=w360, "Address"="10.0.0.100", "Port"=w362) -> (reference out=w359:refnum<k7>, error out=w358:errorcluster)  [unwired: 1 in, 3 out]
          }
        }
      }
      frame "Verify connection" {
        n166 = invoke class="IAsyncChannel" method="GetFirmwareVersion"(reference=w373, error in=w372, "CallType"=u64 0, "pWait"=variant) -> (reference out=w370:refnum<k7>, error out=w366:errorcluster, "GetFirmwareVersion"=w375:string)  [unwired: 1 in, 2 out]
        "FirmwareVersion" <- w375
        n167 = Empty String/Path?(string/path=w375) -> (empty?=w374:bool)
        n168 = Not(x=w374) -> (.not. x?=w371:bool)
        n169 = case shown="False" w371 {
          selector: w371 -> [w378 w401]
          tunnel: w366 -> [w382 w388]
          tunnel: w370 -> [w380 w386]
          tunnel: [w381 w385] -> w367
          tunnel: [w380 w384] -> w369
          tunnel: [T10."Running" T10."Running"] -> w368
          frame False {
            n170 = local write "Connected"(w378) -> ()
            n171 = property on="Connected" class="Bool (strict)"(error in=w382, "Value"=w378) -> (error out=w381:errorcluster)  [unwired: 1 in, 1 out]
            n172 = property on="Enable y-axis" class="Bool (strict)"("Value"=w378) -> ()  [unwired: 2 in, 2 out]
            n173 = property on="Enable z-axis" class="Bool (strict)"("Value"=w378) -> ()  [unwired: 2 in, 2 out]
            n174 = property on="Enable x-axis" class="Bool (strict)"("Value"=w378) -> ()  [unwired: 2 in, 2 out]
          }
          frame True {
            w393 = TRUE ("Boolean")
            w390 = u16 0 items=["X", "Y", "Z"] ("Axes Select")
            w392 = TRUE ("Boolean")
            w389 = u16 1 items=["X", "Y", "Z"] ("Axes Select")
            w391 = TRUE ("Boolean")
            w387 = u16 2 items=["X", "Y", "Z"] ("Axes Select")
            # "Activating stage"
            n175 = call "Stage_enable.vi"("error in (no error)"=w388, "ON=true, OFF = false"=w391, "Axes Select"=w387, "reference"=w386) -> ("error out"=w396:errorcluster, "reference out"=w394:refnum<k7>)  [unwired: 6 in]
            n176 = property on="Enable z-axis" class="Bool (strict)"(error in=w396, "Value"=w391) -> (error out=w397:errorcluster)  [unwired: 1 in, 1 out]
            n177 = call "Stage_enable.vi"("error in (no error)"=w397, "ON=true, OFF = false"=w392, "Axes Select"=w389, "reference"=w394) -> ("error out"=w398:errorcluster, "reference out"=w395:refnum<k7>)  [unwired: 6 in]
            n178 = property on="Enable y-axis" class="Bool (strict)"(error in=w398, "Value"=w392) -> (error out=w399:errorcluster)  [unwired: 1 in, 1 out]
            n179 = call "Stage_enable.vi"("error in (no error)"=w399, "ON=true, OFF = false"=w393, "Axes Select"=w390, "reference"=w395) -> ("error out"=w400:errorcluster, "reference out"=w384:refnum<k7>)  [unwired: 6 in]
            n180 = property on="Enable x-axis" class="Bool (strict)"(error in=w400, "Value"=w393) -> (error out=w385:errorcluster)  [unwired: 1 in, 1 out]
            "Connected" <- w401
          }
        }
      }
      frame "Running", Default {
        # "In the running loop it is checking the position of the stage and listening for events \nlike a button has been pressed and then execute the corresponding action."
        # "Initialization, Running or closing case selector"
        n181 = local read "DAQ Setup"() -> (w402:enum16{"Test setup", "Microscope"})
        n182 = case shown="\"Microscope\"" w402 {
          tunnel: w408 -> [w413 w418]
          tunnel: w407 -> [w412 w417]
          tunnel: [w413 w416] -> w405
          tunnel: [w412 w415] -> w404
          frame "Test setup", Default {
          }
          frame "Microscope" {
            n183 = call "get_stage_position.vi"("error IN"=w417, "reference IN"=w418) -> ("error OUT"=w415:errorcluster, "Stage position OUT"=→"Stage position":T1, "reference OUT"=w416:refnum<k7>)  [unwired: 7 in]
          }
        }
        n184 = event shown="[15] \"Sawtooth generator\": Value Change" {
          selector: _ -> [_ _ _ _ _ _ _ _ _ _ _ _ _ _ _ _ _ _]
          dyn-events: _ -> [_ _ _ _ _ _ _ _ _ _ _ _ _ _ _ _ _ _]
          timeout: 20 -> [_ _ _ _ _ _ _ _ _ _ _ _ _ _ _ _ _ _]
          tunnel: w408 -> [_ w423 w488 w504 _ _ w571 _ _ w590 w639 _ _ _ _ _ w721 _]
          tunnel: w407 -> [_ w422 w487 w503 _ _ w570 _ _ w589 w640 _ _ _ _ _ w722 _]
          tunnel: [_ _ _ _ _ _ w576 _ _ _ _ _ _ _ _ _ _ _] -> w409
          event Timeout {
            n185 = event-data() -> ()  [unwired: 1 in, 3 out]
          }
          event "Calibrate home": Value Change {
            n186 = event-data() -> ()  [unwired: 1 in, 6 out]
            n187 = while {
              shift-right: [w424] -> _
              shift-left: T11."Turn off X and Y" -> [w425]
              shift-right: [w428] -> _
              shift-left: w423 -> [w430]
              shift-right: [w427] -> _
              shift-left: w422 -> [w429]
              stop <- w426 stop-if-true
              n188 = case shown="\"Manually move stage 2\"" w425 {
                tunnel: w430 -> [w435 w447 w454 w471 w476]
                tunnel: w429 -> [w434 w446 w453 w469 w475]
                tunnel: [w433 w447 w452 w471 w474] -> w428
                tunnel: [w432 w446 w451 w468 w473] -> w427
                tunnel: [_ _ _ _ TRUE] -> w426
                tunnel: [T11."Manually move stage 1" w445 T11."Enable Home button" T11."Activate X and Y" _] -> w424
                frame "Turn off X and Y", Default {
                  w439 = FALSE ("ON=true, OFF = false")
                  w438 = u16 1 items=["X", "Y", "Z"] ("Axes Select")
                  w436 = u16 0 items=["X", "Y", "Z"] ("Axes Select")
                  n189 = call "Stage_enable.vi"("error in (no error)"=w434, "ON=true, OFF = false"=FALSE, "Axes Select"=w436, "reference"=w435) -> ("error out"=w441:errorcluster, "reference out"=w442:refnum<k7>)  [unwired: 6 in]
                  n190 = call "Stage_enable.vi"("error in (no error)"=w441, "ON=true, OFF = false"=w439, "Axes Select"=w438, "reference"=w442) -> ("error out"=w443:errorcluster, "reference out"=w433:refnum<k7>)  [unwired: 6 in]
                  n191 = property on="Enable x-axis" class="Bool (strict)"(error in=w443, "Value"=w439) -> (error out=w444:errorcluster)  [unwired: 1 in, 1 out]
                  n192 = property on="Enable y-axis" class="Bool (strict)"(error in=w444, "Value"=FALSE) -> (error out=w432:errorcluster)  [unwired: 1 in, 1 out]
                }
                frame "Manually move stage 1" {
                  n193 = call "Display Message to move stage"() -> ("OK"=w448:bool)  [unwired: 10 in, 1 out]
                  n194 = case shown="True" w448 {
                    tunnel: [_ T11."Manually move stage 2"] -> w445
                    frame False {
                    }
                    frame True {
                    }
                  }
                }
                frame "Manually move stage 2" {
                  n195 = call "Display Message to move stage"() -> ("OK"=w458:bool)  [unwired: 10 in, 1 out]
                  n196 = call "get_stage_position.vi"("error IN"=w453, "reference IN"=w454) -> ("error OUT"=w456:errorcluster, "Stage position OUT"=w455:T1, "reference OUT"=w457:refnum<k7>)  [unwired: 7 in]
                  "Stage position OUT" <- w455
                  n197 = case shown="True" w458 {
                    tunnel: w455 -> [_ w466]
                    tunnel: w457 -> [w460 w465]
                    tunnel: w456 -> [w459 w464]
                    tunnel: [w460 w462] -> w452
                    tunnel: [w459 w461] -> w451
                    frame False {
                    }
                    frame True {
                      n198 = call "get_stage_position.vi"("error IN"=w464, "reference IN"=w465) -> ("error OUT"=w461:errorcluster, "Stage position OUT"=w463:T1, "reference OUT"=w462:refnum<k7>)  [unwired: 7 in]
                      "Stage position OUT 2" <- w463
                      n199 = call "Stage update boundary.vi"("Stage position 2"=w463, "Stage position 1"=w466) -> ()  [unwired: 10 in]
                    }
                  }
                }
                frame "Enable Home button" {
                  n200 = property on="Move Home" class="Bool (strict)"(error in=w469, "Visible"=TRUE) -> (error out=w468:errorcluster)  [unwired: 1 in, 1 out]
                }
                frame "Activate X and Y" {
                  w480 = TRUE ("ON=true, OFF = false")
                  w479 = u16 1 items=["X", "Y", "Z"] ("Axes Select")
                  w477 = u16 0 items=["X", "Y", "Z"] ("Axes Select")
                  n201 = call "Stage_enable.vi"("error in (no error)"=w475, "ON=true, OFF = false"=TRUE, "Axes Select"=w477, "reference"=w476) -> ("error out"=w482:errorcluster, "reference out"=w483:refnum<k7>)  [unwired: 6 in]
                  n202 = call "Stage_enable.vi"("error in (no error)"=w482, "ON=true, OFF = false"=w480, "Axes Select"=w479, "reference"=w483) -> ("error out"=w484:errorcluster, "reference out"=w474:refnum<k7>)  [unwired: 6 in]
                  n203 = property on="Enable x-axis" class="Bool (strict)"(error in=w484, "Value"=w480) -> (error out=w485:errorcluster)  [unwired: 1 in, 1 out]
                  n204 = property on="Enable y-axis" class="Bool (strict)"(error in=w485, "Value"=TRUE) -> (error out=w473:errorcluster)  [unwired: 1 in, 1 out]
                }
              }
            }
          }
          event "Move Home": Value Change {
            n205 = event-data() -> ("NewVal"=w486:bool)  [unwired: 1 in, 5 out]
            n206 = case shown="False" w486 {
              tunnel: w488 -> [_ w502]
              tunnel: w487 -> [_ w501]
              frame False {
              }
              frame True {
                n207 = global read "Global stage boundaries.vi" "Stage boundary positions"() -> (w500:T13)
                n208 = Unbundle By Name(w500) -> ("X lower bound"=w496:dbl, "Y lower bound"=w493:dbl, "Y upper bound"=w492:dbl)
                n209 = Add(x=w493, y=w492) -> (x+y=w491:dbl)
                n210 = Add(x=1.0, y=w496) -> (x+y=w494:dbl)
                n211 = Divide(x=w491, y=2.0) -> (x/y=w489:dbl)
                n212 = local read "Stage position"() -> (w498:T1)
                n213 = Bundle By Name(cluster=w498, "X Position"=w494, "Y Position"=w489, "Z Position"=0.0) -> (w499:T1)
                n214 = call "Stage_move_to_destination.vi"("reference IN"=w502, "Stage position IN"=w499, "error IN"=w501) -> ()  [unwired: 9 in, 4 out]
              }
            }
          }
          event Value Change {
            n215 = event-data() -> ("CtlRef"=w507:refnum<vi>, "NewVal"=w505:bool)  [unwired: 1 in, 4 out]
            n216 = property class="Bool (strict)"(reference=w507) -> ("Label.Text"=w506:string)  [unwired: 1 in, 2 out]
            n217 = case shown="\"Enable x-axis\"" w506 {
              tunnel: w505 -> [_ w508 w512 w516]
              tunnel: w504 -> [_ w509 w514 w518]
              tunnel: w503 -> [_ w510 w513 w517]
              frame Default {
              }
              frame "Enable y-axis" {
                w511 = u16 1 items=["X", "Y", "Z"] ("Axes Select")
                n218 = call "Stage_enable.vi"("error in (no error)"=w510, "ON=true, OFF = false"=w508, "Axes Select"=w511, "reference"=w509) -> ()  [unwired: 6 in, 2 out]
              }
              frame "Enable z-axis" {
                w515 = u16 2 items=["X", "Y", "Z"] ("Axes Select")
                n219 = call "Stage_enable.vi"("error in (no error)"=w513, "ON=true, OFF = false"=w512, "Axes Select"=w515, "reference"=w514) -> ()  [unwired: 6 in, 2 out]
              }
              frame "Enable x-axis" {
                w519 = u16 0 items=["X", "Y", "Z"] ("Axes Select")
                n220 = call "Stage_enable.vi"("error in (no error)"=w517, "ON=true, OFF = false"=w516, "Axes Select"=w519, "reference"=w518) -> ()  [unwired: 6 in, 2 out]
              }
            }
          }
          event Value Change {
            # "Enabling/disabling control keys depending on the same step size buttom"
            n221 = event-data() -> ("NewVal"=w522:bool)  [unwired: 1 in, 5 out]
            n222 = local read "Stage control"() -> (w521:T2)
            n223 = Unbundle By Name(w521) -> ("Global step size (um)"=w520:dbl)
            n224 = case shown="True" w522 {
              tunnel: w520 -> [_ w534]
              frame False {
                n225 = property on="Global step size (um)" class="DigNum (strict)"("DisabledEnum"=T12."Disabled and Grayed Out" ("Disabled")) -> (error out=w523:errorcluster)  [unwired: 2 in, 1 out]
                n226 = property on="X Step Size(um)" class="DigNum (strict)"(error in=w523, "DisabledEnum"=T12."Enabled" ("Disabled")) -> (error out=w527:errorcluster)  [unwired: 1 in, 1 out]
                n227 = property on="Y Step Size(um)" class="DigNum (strict)"(error in=w527, "DisabledEnum"=T12."Enabled" ("Disabled")) -> (error out=w525:errorcluster)  [unwired: 1 in, 1 out]
                n228 = property on="Z step size (um)" class="DigNum (strict)"(error in=w525, "DisabledEnum"=T12."Enabled" ("Disabled")) -> ()  [unwired: 1 in, 2 out]
              }
              frame True {
                n229 = property on="X Step Size(um)" class="DigNum (strict)"("Value"=w534) -> (error out=w533:errorcluster)  [unwired: 2 in, 1 out]
                n230 = property on="Global step size (um)" class="DigNum (strict)"("DisabledEnum"=T12."Enabled" ("Disabled")) -> (error out=w530:errorcluster)  [unwired: 2 in, 1 out]
                n231 = property on="Y Step Size(um)" class="DigNum (strict)"(error in=w533, "Value"=w534) -> (error out=w532:errorcluster)  [unwired: 1 in, 1 out]
                n232 = property on="X Step Size(um)" class="DigNum (strict)"(error in=w530, "DisabledEnum"=T12."Disabled and Grayed Out" ("Disabled")) -> (error out=w537:errorcluster)  [unwired: 1 in, 1 out]
                n233 = property on="Z step size (um)" class="DigNum (strict)"(error in=w532, "Value"=w534) -> ()  [unwired: 1 in, 2 out]
                n234 = property on="Y Step Size(um)" class="DigNum (strict)"(error in=w537, "DisabledEnum"=T12."Disabled and Grayed Out" ("Disabled")) -> (error out=w535:errorcluster)  [unwired: 1 in, 1 out]
                n235 = property on="Z step size (um)" class="DigNum (strict)"(error in=w535, "DisabledEnum"=T12."Disabled and Grayed Out" ("Disabled")) -> ()  [unwired: 1 in, 2 out]
              }
            }
          }
          event "Tab Control": Value Change {
            n236 = event-data() -> ("NewVal"=w540:enum32{"Manual setup", "Acquisition", "Debug"})  [unwired: 1 in, 5 out]
            n237 = case shown="\"Acquisition\"" w540 {
              frame "Manual setup", Default {
                w543 = T12."Enabled" ("Disabled")
                n238 = global write "Global stop DAQ.vi" "Global stop DAQ"(TRUE ("Global stop DAQ")) -> ()
                n239 = property on="Voice coil calibration file" class="Path"() -> ("Value"=w541:path)  [unwired: 2 in, 2 out]
                n240 = Bundle("", 0.0) -> (w551:cluster{string, dbl})  [unwired: 1 in]
                n241 = local write "Voice coil \ncontrol mode"(T4."Manual" ("Voice coil \ncontrol mode")) -> ()
                n242 = Obtain Queue(name (unnamed)="DAQ queue", element data type=w551) -> (queue out=w550:refnum<queue>, error out=w549:errorcluster)  [unwired: 3 in, 1 out]
                n243 = call "Get_file_1st_element.vi"("File Path"=w541) -> ("First element"=w542:dbl)  [unwired: 10 in]
                n244 = Bundle("Manual", "First element"=w542) -> (w548:cluster{string, "First element":dbl})  [unwired: 1 in]
                n245 = Enqueue Element(queue=w550, element=w548, error in (no error)=w549) -> ()  [unwired: 1 in, 3 out]
                n246 = property on="Voice coil voltage output [V]" class="DigNum (strict)"("DisabledEnum"=w543) -> ()  [unwired: 2 in, 2 out]
                n247 = property on="Voice coil voltage slider" class="Slide (strict)"("DisabledEnum"=w543) -> ()  [unwired: 2 in, 2 out]
              }
              frame "Acquisition" {
                # "Stopping DAQ before allowing acquisition again"
                n248 = flat-sequence {
                  frame #0 {
                    n249 = global write "Global stop DAQ.vi" "Global stop DAQ"(TRUE ("Global stop DAQ")) -> ()
                    n250 = Wait (ms)(milliseconds to wait=u32 500) -> ()  [unwired: 1 out]
                  }
                  frame #1 {
                    n251 = global write "Global stop DAQ.vi" "Global stop DAQ"(FALSE ("Global stop DAQ")) -> ()
                  }
                }
              }
            }
          }
          event Value Change {
            n252 = event-data() -> ("NewVal"=w576:bool)  [unwired: 1 in, 5 out]
            n253 = Bundle("", 0.0) -> (w569:cluster{string, dbl})  [unwired: 1 in]
            n254 = Bundle("element"="stop", "reference OUT"=w571, "error OUT"=w570) -> (w558:T9)  [unwired: 1 in]
            n255 = local read "output cluster"() -> (w559:T9)
            n256 = Obtain Queue(name (unnamed)="DAQ queue", element data type=w569) -> (queue out=w565:refnum<queue>, error out=w564:errorcluster)  [unwired: 3 in, 1 out]
            n257 = Obtain Queue(name (unnamed)="Acquisition Handler", element data type=w559) -> (queue out=w574:refnum<queue>, error out=w573:errorcluster)  [unwired: 3 in, 1 out]
            n258 = Bundle("stop", 0.0) -> (w561:cluster{string, dbl})  [unwired: 1 in]
            n259 = Enqueue Element(queue=w574, element=w558, error in (no error)=w573) -> ()  [unwired: 1 in, 3 out]
            n260 = Enqueue Element(queue=w565, element=w561, error in (no error)=w564) -> ()  [unwired: 1 in, 3 out]
            n261 = global write "Global stop DAQ.vi" "Global stop DAQ"(TRUE ("Global stop DAQ")) -> ()
            n262 = global write "Global stop.vi" "Global stop"(TRUE ("Global stop")) -> ()
          }
          event "Abort acquisition": Value Change {
            n263 = event-data() -> ("NewVal"=w577:bool)  [unwired: 1 in, 5 out]
            n264 = case shown="True" w577 {
              frame False {
              }
              frame True {
                n265 = call "Display Message to User"() -> ("Yes"=w578:bool)  [unwired: 10 in, 1 out]
                n266 = case shown="True" w578 {
                  frame False {
                  }
                  frame True {
                    w581 = "CommandSequenceHandler" ("name (unnamed)")
                    n267 = flat-sequence {
                      frame #0 {
                        n268 = global write "Global Z-stack acquistion finished flag.vi" "Z-stack acquisition finished flag"(TRUE ("Z-stack acquisition finished flag")) -> ()
                        n269 = global write "Global stop DAQ.vi" "Global stop DAQ"(TRUE ("Global stop DAQ")) -> ()
                      }
                      frame #1 {
                        n270 = Wait (ms)(milliseconds to wait=u32 200) -> ()  [unwired: 1 out]
                      }
                      frame #2 {
                        n271 = global write "Global stop DAQ.vi" "Global stop DAQ"(FALSE ("Global stop DAQ")) -> ()
                      }
                    }
                    n272 = Obtain Queue(name (unnamed)=w581, element data type=w581) -> (queue out=w580:refnum<queue>, error out=w579:errorcluster)  [unwired: 3 in, 1 out]
                    n273 = Flush Queue(queue=w580, error in (no error)=w579) -> ()  [unwired: 3 out]
                  }
                }
              }
            }
          }
          event Value Change {
            # "Update the XYZ step sizes to be that of the global step size"
            n274 = event-data() -> ("NewVal"=w588:dbl)  [unwired: 1 in, 5 out]
            n275 = property on="X Step Size(um)" class="DigNum (strict)"("Value"=w588) -> (error out=w587:errorcluster)  [unwired: 2 in, 1 out]
            n276 = property on="Y Step Size(um)" class="DigNum (strict)"(error in=w587, "Value"=w588) -> (error out=w586:errorcluster)  [unwired: 1 in, 1 out]
            n277 = property on="Z step size (um)" class="DigNum (strict)"(error in=w586, "Value"=w588) -> ()  [unwired: 1 in, 2 out]
          }
          event Value Change {
            n278 = event-data() -> ("CtlRef"=w592:refnum<vi>, "NewVal"=w591:bool)  [unwired: 1 in, 4 out]
            n279 = case shown="True" w591 {
              tunnel: w592 -> [_ w597]
              tunnel: w590 -> [_ w594]
              tunnel: w589 -> [_ w593]
              frame False {
              }
              frame True {
                n280 = property class="Bool (strict)"(reference=w597) -> ("Label.Text"=w596:string)  [unwired: 1 in, 2 out]
                n281 = local read "Stage control"() -> (w595:T2)
                n282 = case shown="Default" w596 {
                  tunnel: w595 -> [w603 w609 w615 w621 w627 w633 _]
                  tunnel: w594 -> [w602 w608 w614 w620 w626 w632 _]
                  tunnel: w593 -> [w601 w607 w613 w619 w625 w631 _]
                  frame "Left" {
                    w599 = u16 1 items=["X", "Y", "Z"] ("Axes Select")
                    n283 = Unbundle By Name(w603) -> ("Y Step Size(um)"=w598:dbl)
                    n284 = call "Stage_move_axis.vi"("Direction true means positive increment"=FALSE, "error in (no error)"=w601, "Distance micrometer"=w598, "Axes Select"=w599, "reference IN"=w602) -> ()  [unwired: 5 in, 2 out]
                  }
                  frame "Right" {
                    w605 = u16 1 items=["X", "Y", "Z"] ("Axes Select")
                    n285 = Unbundle By Name(w609) -> ("Y Step Size(um)"=w604:dbl)
                    n286 = call "Stage_move_axis.vi"("Direction true means positive increment"=TRUE, "error in (no error)"=w607, "Distance micrometer"=w604, "Axes Select"=w605, "reference IN"=w608) -> ()  [unwired: 5 in, 2 out]
                  }
                  frame "Up" {
                    w611 = u16 0 items=["X", "Y", "Z"] ("Axes Select")
                    n287 = Unbundle By Name(w615) -> ("X Step Size(um)"=w610:dbl)
                    n288 = call "Stage_move_axis.vi"("Direction true means positive increment"=TRUE, "error in (no error)"=w613, "Distance micrometer"=w610, "Axes Select"=w611, "reference IN"=w614) -> ()  [unwired: 5 in, 2 out]
                  }
                  frame "Down" {
                    w617 = u16 0 items=["X", "Y", "Z"] ("Axes Select")
                    n289 = Unbundle By Name(w621) -> ("X Step Size(um)"=w616:dbl)
                    n290 = call "Stage_move_axis.vi"("Direction true means positive increment"=FALSE, "error in (no error)"=w619, "Distance micrometer"=w616, "Axes Select"=w617, "reference IN"=w620) -> ()  [unwired: 5 in, 2 out]
                  }
                  frame "Z Up" {
                    w623 = u16 2 items=["X", "Y", "Z"] ("Axes Select")
                    n291 = Unbundle By Name(w627) -> ("Z step size (um)"=w622:dbl)
                    n292 = call "Stage_move_axis.vi"("Direction true means positive increment"=TRUE, "error in (no error)"=w625, "Distance micrometer"=w622, "Axes Select"=w623, "reference IN"=w626) -> ()  [unwired: 5 in, 2 out]
                  }
                  frame "Z Down" {
                    w629 = u16 2 items=["X", "Y", "Z"] ("Axes Select")
                    n293 = Unbundle By Name(w633) -> ("Z step size (um)"=w628:dbl)
                    n294 = call "Stage_move_axis.vi"("Direction true means positive increment"=FALSE, "error in (no error)"=w631, "Distance micrometer"=w628, "Axes Select"=w629, "reference IN"=w632) -> ()  [unwired: 5 in, 2 out]
                  }
                  frame Default {
                  }
                }
              }
            }
          }
          event Value Change {
            n295 = event-data() -> ()  [unwired: 1 in, 6 out]
            n296 = property on="Destination" class="Clust (strict)"(error in=w640) -> (error out=w637:errorcluster, "Value"=w638:T1)  [unwired: 1 in, 1 out]
            n297 = call "Stage_move_to_destination.vi"("reference IN"=w639, "Stage position IN"=w638, "Number of times it should see if destination is achieved"=3.0, "milliseconds to wait"=u32 1000, "error IN"=w637) -> ("Stage position OUT"=w636:T1)  [unwired: 7 in, 3 out]
            n298 = local write "Stage position"(w636) -> ()
          }
          event "Voice coil \ncontrol mode": Value Change {
            n299 = event-data() -> ("NewVal"=w647:T4)  [unwired: 1 in, 5 out]
            n300 = case shown="\"Saw tooth function\"" w647 {
              tunnel: [w650 w655 w660] -> w648
              frame "Manual", Default {
                w653 = T12."Enabled" ("Disabled")
                n301 = global write "Global stop DAQ.vi" "Global stop DAQ"(TRUE ("Global stop DAQ")) -> ()
                n302 = property on="Voice coil voltage output [V]" class="DigNum (strict)"("DisabledEnum"=w653) -> ()  [unwired: 2 in, 2 out]
                n303 = property on="Voice coil voltage slider" class="Slide (strict)"("DisabledEnum"=w653) -> ()  [unwired: 2 in, 2 out]
                n304 = Bundle("Manual", 0.0) -> (w650:cluster{string, dbl})  [unwired: 1 in]
              }
              frame "Saw tooth function" {
                w658 = T12."Disabled and Grayed Out" ("Disabled")
                n305 = global write "Global stop DAQ.vi" "Global stop DAQ"(TRUE ("Global stop DAQ")) -> ()
                n306 = property on="Voice coil voltage output [V]" class="DigNum (strict)"("DisabledEnum"=w658) -> ()  [unwired: 2 in, 2 out]
                n307 = property on="Voice coil voltage slider" class="Slide (strict)"("DisabledEnum"=w658) -> ()  [unwired: 2 in, 2 out]
                n308 = Bundle("sawtooth", 0.0) -> (w655:cluster{string, dbl})  [unwired: 1 in]
              }
              frame "From file" {
                w663 = T12."Disabled and Grayed Out" ("Disabled")
                n309 = global write "Global stop DAQ.vi" "Global stop DAQ"(TRUE ("Global stop DAQ")) -> ()
                n310 = property on="Voice coil voltage output [V]" class="DigNum (strict)"("DisabledEnum"=w663) -> ()  [unwired: 2 in, 2 out]
                n311 = property on="Voice coil voltage slider" class="Slide (strict)"("DisabledEnum"=w663) -> ()  [unwired: 2 in, 2 out]
                n312 = Bundle("signal", 0.0) -> (w660:cluster{string, dbl})  [unwired: 1 in]
              }
            }
            n313 = Bundle("", 0.0) -> (w643:cluster{string, dbl})  [unwired: 1 in]
            n314 = Obtain Queue(name (unnamed)="DAQ queue", element data type=w643) -> (queue out=w642:refnum<queue>, error out=w641:errorcluster)  [unwired: 3 in, 1 out]
            n315 = Enqueue Element(queue=w642, element=w648, error in (no error)=w641) -> ()  [unwired: 1 in, 3 out]
          }
          event Value Change {
            n316 = event-data() -> ("CtlRef"=w666:refnum<vi>, "NewVal"=w665:path)  [unwired: 1 in, 4 out]
            n317 = property class="Path"(reference=w666) -> ("Label.Text"=w664:string)  [unwired: 1 in, 2 out]
            n318 = case shown="\"Voice coil calibration file\"" w664 {
              tunnel: w665 -> [_ w668 w670]
              frame "False", Default {
              }
              frame "Voice coil calibration file" {
                n319 = local read "Voice coil function generation"() -> (w669:T5)
                n320 = Bundle By Name(cluster=w669, "File to read"=w668) -> (w667:T5)
                n321 = local write "Voice coil function generation"(w667) -> ()
              }
              frame "File to read" {
                n322 = property on="Voice coil calibration file" class="Path"("Value"=w670) -> ()  [unwired: 2 in, 2 out]
              }
            }
          }
          event Value Change {
            n323 = event-data() -> ()  [unwired: 1 in, 6 out]
            n324 = Bundle("", 0.0) -> (w677:cluster{string, dbl})  [unwired: 1 in]
            n325 = Obtain Queue(name (unnamed)="DAQ queue", element data type=w677) -> (queue out=w676:refnum<queue>, error out=w675:errorcluster)  [unwired: 3 in, 1 out]
            n326 = global write "Global stop DAQ.vi" "Global stop DAQ"(TRUE ("Global stop DAQ")) -> ()
            n327 = local read "Voice coil \ncontrol mode"() -> (w673:T4)
            n328 = Bundle("AOTF", 0.0) -> (w681:cluster{string, dbl})  [unwired: 1 in]
            n329 = Enqueue Element(queue=w676, element=w681, error in (no error)=w675) -> (queue out=w672:refnum<queue>, error out=w671:errorcluster)  [unwired: 1 in, 1 out]
            n330 = case shown="\"Saw tooth function\"" w673 {
              tunnel: w672 -> [_ w685 w690]
              tunnel: w671 -> [_ w684 w689]
              frame "Manual", Default {
              }
              frame "From file" {
                n331 = Bundle("signal", 0.0) -> (w688:cluster{string, dbl})  [unwired: 1 in]
                n332 = Enqueue Element(queue=w685, element=w688, error in (no error)=w684) -> ()  [unwired: 1 in, 3 out]
              }
              frame "Saw tooth function" {
                n333 = Bundle("sawtooth", 0.0) -> (w693:cluster{string, dbl})  [unwired: 1 in]
                n334 = Enqueue Element(queue=w690, element=w693, error in (no error)=w689) -> ()  [unwired: 1 in, 3 out]
              }
            }
          }
          event "Voice coil voltage slider", "Voice coil voltage output [V]": Value Change {
            n335 = event-data() -> ("CtlRef"=w697:refnum<vi>, "NewVal"=w695:dbl)  [unwired: 1 in, 4 out]
            n336 = property class="Num"(reference=w697) -> ("Label.Text"=w696:string)  [unwired: 1 in, 2 out]
            n337 = case shown="\"Voice coil voltage slider\"" w696 {
              tunnel: w695 -> [_ w706 w707]
              tunnel: [_ w706 w707] -> w694
              frame "False", Default {
              }
              frame "Voice coil voltage output" {
                n338 = property on="Voice coil voltage slider" class="Slide (strict)"("Value"=w706) -> ()  [unwired: 2 in, 2 out]
              }
              frame "Voice coil voltage slider" {
                n339 = property on="Voice coil voltage output [V]" class="DigNum (strict)"("Value"=w707) -> ()  [unwired: 2 in, 2 out]
              }
            }
            n340 = Bundle("", 0.0) -> (w700:cluster{string, dbl})  [unwired: 1 in]
            n341 = Obtain Queue(name (unnamed)="DAQ queue", element data type=w700) -> (queue out=w699:refnum<queue>, error out=w698:errorcluster)  [unwired: 3 in, 1 out]
            n342 = Bundle("String"="Manual", "NewVal"=w694) -> (w704:cluster{"String":string, "NewVal":dbl})  [unwired: 1 in]
            n343 = Enqueue Element(queue=w699, element=w704, error in (no error)=w698) -> ()  [unwired: 1 in, 3 out]
          }
          event Value Change {
            n344 = event-data() -> ()  [unwired: 1 in, 6 out]
            n345 = local read "Voice coil \ncontrol mode"() -> (w708:T4)
            n346 = case shown="\"Saw tooth function\"" w708 {
              frame "Manual", Default {
              }
              frame "Saw tooth function" {
                n347 = flat-sequence {
                  frame #0 {
                    n348 = global write "Global stop DAQ.vi" "Global stop DAQ"(TRUE ("Global stop DAQ")) -> ()
                    n349 = Wait (ms)(milliseconds to wait=u32 500) -> ()  [unwired: 1 out]
                  }
                  frame #1 {
                    w711 = 0.0
                    n350 = Bundle("", w711) -> (w714:cluster{string, dbl})  [unwired: 1 in]
                    n351 = Obtain Queue(name (unnamed)="DAQ queue", element data type=w714) -> (queue out=w713:refnum<queue>, error out=w712:errorcluster)  [unwired: 3 in, 1 out]
                    n352 = Bundle("String"="sawtooth", w711) -> (w717:cluster{"String":string, dbl})  [unwired: 1 in]
                    n353 = Enqueue Element(queue=w713, element=w717, error in (no error)=w712) -> ()  [unwired: 1 in, 3 out]
                  }
                }
              }
            }
          }
          event Value Change {
            n354 = event-data() -> ("CtlRef"=w720:refnum<vi>, "NewVal"=w719:bool)  [unwired: 1 in, 4 out]
            n355 = case shown="True" w719 {
              tunnel: w722 -> [_ w726]
              tunnel: w721 -> [_ w725]
              tunnel: w720 -> [_ w724]
              frame False {
              }
              frame True {
                n356 = property class="Bool (strict)"(reference=w724) -> ("Label.Text"=w723:string)  [unwired: 1 in, 2 out]
                n357 = case shown="\"Acquire XY-tiling\"" w723 {
                  tunnel: w726 -> [_ w729 _ _]
                  tunnel: w725 -> [_ w728 _ _]
                  frame "False", Default {
                  }
                  frame "Acquire Z-stack" {
                    n358 = Bundle("element"="acquire Zstack", "reference OUT"=w728, "error OUT"=w729) -> (w727:T9)  [unwired: 1 in]
                    n359 = local write "output cluster"(w727) -> ()
                    n360 = Obtain Queue(name (unnamed)="Acquisition Handler", element data type=w727) -> (queue out=w732:refnum<queue>, error out=w731:errorcluster)  [unwired: 3 in, 1 out]
                    n361 = Enqueue Element(queue=w732, element=w727, error in (no error)=w731) -> ()  [unwired: 1 in, 3 out]
                  }
                  frame "Acquire" {
                    w737 = "CommandSequenceHandler" ("name (unnamed)")
                    n362 = property on="typedef_laser_order_control" class="Clust (strict)" props=["Value"]() -> ()  [unwired: 2 in, 3 out]
                    n363 = Obtain Queue(name (unnamed)=w737, element data type=w737) -> (queue out=w736:refnum<queue>, error out=w735:errorcluster)  [unwired: 3 in, 1 out]
                    n364 = Enqueue Element(queue=w736, element="Start sequence", error in (no error)=w735) -> ()  [unwired: 1 in, 3 out]
                  }
                  frame "Acquire XY-tiling" {
                    w741 = "CommandSequenceHandler" ("name (unnamed)")
                    n365 = Obtain Queue(name (unnamed)=w741, element data type=w741) -> (queue out=w740:refnum<queue>, error out=w739:errorcluster)  [unwired: 3 in, 1 out]
                    n366 = Enqueue Element(queue=w740, element="Start sequence", error in (no error)=w739) -> ()  [unwired: 1 in, 3 out]
                  }
                }
              }
            }
          }
          event Value Change {
            n367 = event-data() -> ("CtlRef"=w745:refnum<vi>, "NewVal"=w743:dbl)  [unwired: 1 in, 4 out]
            n368 = property class="DigNum (strict)"(reference=w745) -> ("Label.Text"=w744:string)  [unwired: 1 in, 2 out]
            n369 = case shown="\"Percentage overlap\"" w744 {
              tunnel: w743 -> [_ w751 w757]
              tunnel: "FOV (um)" -> [_ w749 w752]
              frame "False", Default {
              }
              frame "Step size X and Y (um)" {
                n370 = Subtract(x=w749, y=w751) -> (x-y=w750:dbl)
                n371 = Divide(x=w750, y=w749) -> (x/y=w748:dbl)
                n372 = Multiply(x=w748, y=100.0) -> (x*y=w746:dbl)
                n373 = property on="Percentage overlap" class="DigNum (strict)"("Value"=w746) -> ()  [unwired: 2 in, 2 out]
              }
              frame "Percentage overlap" {
                n374 = Subtract(x=100.0, y=w757) -> (x-y=w755:dbl)
                n375 = Divide(x=w755, y=100.0) -> (x/y=w753:dbl)
                n376 = Multiply(x=w752, y=w753) -> (x*y=w754:dbl)
                n377 = property on="Step size X and Y (um)" class="DigNum (strict)"("Value"=w754) -> ()  [unwired: 2 in, 2 out]
              }
            }
          }
        }
        n378 = Bundle("element"="acquire Zstack", "reference OUT"=w405, "error OUT"=w404) -> (→"output cluster":T9)  [unwired: 1 in]
        n379 = case shown="True" w409 {
          tunnel: [T10."Running" T10."Closing"] -> w411
          frame False {
          }
          frame True {
          }
        }
      }
      frame "Closing" {
        n380 = local write "Connected"(FALSE ("Connected")) -> ()
        n381 = invoke class="IAsyncChannel" method="CloseComm"(reference=w760, error in=w759) -> (error out=→"Error out":errorcluster)  [unwired: 1 in, 2 out]
      }
    }
  }
  n382 = while {
    tunnel: w8 -> [w769]
    tunnel: w7 -> [w768]
    stop <- w764 stop-if-true
    n383 = Dequeue Element(queue=w769, error in (no error)=w768) -> (element=w767:cluster{string, dbl})  [unwired: 1 in, 3 out]
    n384 = Unbundle(w767) -> (w765:string, w766:dbl)
    n385 = case shown="\"sawtooth\"" w765 {
      tunnel: w766 -> [_ w775 _ _ _ _]
      tunnel: [_ _ _ _ _ TRUE] -> w764
      frame "0", Default {
      }
      frame "Manual" {
        (unwired) "Voice coil" ("new task name")
        n386 = local read "DAQ Setup"() -> (w772:enum16{"Test setup", "Microscope"})
        n387 = call "DAQ_channel_setup.vi"("Text Ring"=w772) -> ("DAQ channels OUT"=w771:T14)  [unwired: 10 in]
        n388 = Unbundle By Name(w771) -> ("Voice coil analog output"=w770:tag)
        n389 = call <vilib>:"DAQmx Create Task.vi"("auto cleanup"=TRUE, "error in"="error in") -> ("task out"=w786:refnum<k21>, "error out"=w785:errorcluster)  [unwired: 12 in]
        n390 = call-poly <vilib>:"DAQmx Create Virtual Channel.vi"("task in"=w786, "maximum value"=0.6, "minimum value"=-0.6, "physical channels"=w770, "error in"=w785) -> ("task out"=w782:refnum<k21>, "error out"=w781:errorcluster)  [unwired: 9 in]
        n391 = call-poly <vilib>:"DAQmx Write.vi"("task/channels in"=w782, "auto start"=TRUE, "data"=w775, "error in"=w781) -> ("task out"=w777:refnum<k21>, "error out"=w776:errorcluster)  [unwired: 9 in, 1 out]
        n392 = call <vilib>:"DAQmx Stop Task.vi"("task/channels in"=w777, "error in"=w776) -> ("task out"=w778:refnum<k21>, "error out"=w779:errorcluster)  [unwired: 12 in]
        n393 = call <vilib>:"DAQmx Clear Task.vi"("task in"=w778, "error in"=w779) -> ()  [unwired: 13 in, 1 out]
      }
      frame "AOTF" {
        n394 = local read "Laser Toggles"() -> (w788:T3)
        n395 = local read "DAQ Setup"() -> (w787:enum16{"Test setup", "Microscope"})
        n396 = call "AOTF laser control manual.vi"("DAQ setup"=w787, "Laser Toggles"=w788) -> ()  [unwired: 10 in]
      }
      frame "signal" {
        n397 = call "Dac_release_all_lines.vi"("Release all DAQ lines"=FALSE) -> ("error out"=w790:errorcluster)  [unwired: 9 in, 1 out]
        n398 = local read "DAQ Setup"() -> (w789:enum16{"Test setup", "Microscope"})
        n399 = call "Dac_Voice_coil_Camera_trigger.vi"("Voice coil function generation"="Voice coil function generation", "error in"=w790, "DAQ setup"=w789) -> ()  [unwired: 17 in]
      }
      frame "sawtooth" {
        n400 = local read "DAQ Setup"() -> (w796:enum16{"Test setup", "Microscope"})
        n401 = call "DAQ_channel_setup.vi"("Text Ring"=w796) -> ("DAQ channels OUT"=w795:T14)  [unwired: 10 in]
        n402 = Unbundle By Name(w795) -> ("Voice coil analog output"=w794:tag)
        n403 = call "Sawtooth generation VI.vi"("physical channels"=w794, "Sawtooth generator"="Sawtooth generator") -> ()  [unwired: 8 in, 1 out]
      }
      frame "stop" {
      }
    }
  }
  n404 = while {
    tunnel: w4 -> [w806]
    tunnel: w3 -> [w805]
    stop <- w803 stop-if-true
    n405 = Dequeue Element(queue=w806, timeout in ms (-1)=1, error in (no error)=w805) -> (element=w804:string)  [unwired: 3 out]
    n406 = case shown="\"Start sequence\"" w804 {
      frame "False", Default {
      }
      frame "Start sequence" {
        n407 = local read "Acquisition"() -> (w808:T7)
        n408 = property on="Acquisition" class="Clust (strict)"("DisabledEnum"=T12."Disabled" ("Disabled")) -> ()  [unwired: 2 in, 2 out]
        n409 = call "XYZ_sequence_generator_with_flags.vi"("X-direction"="X-direction", "Y-direction"="Y-direction", "Acquisition"=w808) -> ("string array"=w809:string[])  [unwired: 7 in, 1 out]
        n410 = while {
          tunnel: w809 -> [w815]
          stop <- w819 stop-if-true
          n411 = local read "output cluster"() -> (w816:T9)
          n412 = Array Size(array=w815) -> (size(s)=w817:i32)
          "Number of commands" <- w817
          n413 = Obtain Queue(name (unnamed)="Acquisition Handler", element data type=w816) -> (queue out=w821:refnum<queue>, error out=w820:errorcluster)  [unwired: 3 in, 1 out]
          n414 = for {
            N: w817 -> [w827]
            tunnel: w815 -> [w833] mode=indexing
            tunnel: w821 -> [w835]
            tunnel: w820 -> [w834]
            tunnel: [w823] -> w818
            shift-right: [w830] -> _
            shift-left: _ -> [w829]
            i -> [w828]
            stop <- w823 stop-if-true
            n415 = Divide(x=w828, y=w827) -> (x/y=w826:dbl)
            n416 = String Subset(string=w833, length (rest)=4 ("length (rest)")) -> (substring=w832:string)  [unwired: 1 in]
            n417 = Multiply(x=w826, y=100.0) -> (x*y=w824:dbl)
            n418 = case shown="\"False\", Default" w832 {
              tunnel: w835 -> [w845 _ w871 _]
              tunnel: w834 -> [w844 _ w870 _]
              tunnel: w833 -> [w840 w850 w868 w881]
              tunnel: w827 -> [w843 _ _ _]
              tunnel: [w836 _ w864 _] -> w823
              tunnel: w828 -> [w841 _ _ _]
              tunnel: [w840 _ w865 _] -> w830
              tunnel: w829 -> [_ _ _ _]
              frame "False", Default {
                n419 = Increment(x=w841) -> (x+1=w842:i32)
                n420 = local read "output cluster"() -> (w839:T9)
                n421 = Equal?(x=w843, y=w842) -> (x = y?=w836:bool)
                n422 = Unbundle By Name(w839) -> ("reference OUT"=w838:refnum<k7>)
                n423 = Bundle By Name(cluster=w839, "element"=w840, "reference OUT"=w838) -> (w837:T9)
                n424 = Enqueue Element(queue=w845, element=w837, error in (no error)=w844) -> ()  [unwired: 1 in, 3 out]
              }
              frame "MOVE" {
                n425 = local read "DAQ Setup"() -> (w847:enum16{"Test setup", "Microscope"})
                n426 = String Subset(string=w850, offset (0)=4 ("length (rest)")) -> (substring=w848:string)  [unwired: 1 in]
                n427 = case shown="\"Microscope\"" w847 {
                  tunnel: w848 -> [w851 w860]
                  tunnel: [w851 w858] -> w846
                  frame "Test setup", Default {
                  }
                  frame "Microscope" {
                    n428 = local read "Acquisition"() -> (w853:T7)
                    n429 = local read "output cluster"() -> (w857:T9)
                    n430 = local read "Z-stack start position"() -> (w855:T1)
                    n431 = Unbundle By Name(w853) -> ("Step size X and Y (um)"=w859:dbl, "Step size Z (um)"=w852:dbl)
                    n432 = Unbundle By Name(w857) -> ("reference OUT"=w856:refnum<k7>)
                    n433 = call "String_to_move_stage.vi"("reference IN"=w856, "Stage position IN"=w855, "Movement string"=w860, "XY step size (µm)"=w859, "Z step size (µm)"=w852) -> ("String"=w858:string, "error OUT"=w854:errorcluster)  [unwired: 8 in, 1 out]
                    n434 = while {
                      tunnel: w854 -> [_]
                      i -> [w862]
                      stop <- w863 stop-if-true
                      n435 = global read "Global destination achieved.vi" "Global destination achieved"() -> (w863:bool)
                      n436 = Wait (ms)(milliseconds to wait=u32 1) -> ()  [unwired: 1 out]
                      "Numeric 4" <- w862
                    }
                  }
                }
                "String" <- w846
              }
              frame "acqu" {
                n437 = global write "Global Z-stack acquistion finished flag.vi" "Z-stack acquisition finished flag"(FALSE ("Z-stack acquisition finished flag")) -> ()
                n438 = local read "output cluster"() -> (w869:T9)
                n439 = Bundle By Name(cluster=w869, "element"=w868) -> (w867:T9)
                n440 = Enqueue Element(queue=w871, element=w867, error in (no error)=w870) -> ()  [unwired: 1 in, 3 out]
                n441 = while {
                  tunnel: [""] -> w865
                  tunnel: [w872] -> w864
                  i -> [w877]
                  stop <- w873 stop-if-true
                  n442 = global read "Global stop DAQ.vi" "Global stop DAQ"() -> (w872:bool)
                  n443 = global read "Global Z-stack acquistion finished flag.vi" "Z-stack acquisition finished flag"() -> (w874:bool)
                  n444 = Wait (ms)(milliseconds to wait=u32 1) -> ()  [unwired: 1 out]
                  n445 = Or(x=w874, y=w872) -> (x .or. y?=w873:bool)
                  "Numeric 3" <- w877
                }
              }
              frame "WAIT" {
                n446 = String Subset(string=w881, offset (0)=4) -> (substring=w879:string)  [unwired: 1 in]
                n447 = Fract/Exp String To Number(string=w879) -> (number=w878:dbl)  [unwired: 3 in, 1 out]
                "waiting time (ms)" <- w878
                n448 = Wait (ms)(milliseconds to wait=w878) -> ()  [unwired: 1 out]
              }
            }
            n449 = property on="Total progress" class="Slide (strict)"("Value"=w824) -> ()  [unwired: 2 in, 2 out]
            "current position in string array" <- w828
          }
          n450 = global read "Global stop.vi" "Global stop"() -> (w814:bool)
          n451 = global read "Global stop DAQ.vi" "Global stop DAQ"() -> (w812:bool)
          n452 = Or(x=w814, y=w812) -> (x .or. y?=w813:bool)
          n453 = Or(x=w818, y=w813) -> (x .or. y?=w819:bool)
          "string array" <- w815
        }
      }
    }
    n454 = property on="Acquisition" class="Clust (strict)"("DisabledEnum"=T12."Enabled" ("Disabled")) -> ()  [unwired: 2 in, 2 out]
    n455 = property on="Total progress" class="Slide (strict)"("Value"=u8 0) -> ()  [unwired: 2 in, 2 out]
    n456 = global read "Global stop.vi" "Global stop"() -> (w801:bool)
    n457 = Or(x="stop", y=w801) -> (x .or. y?=w803:bool)
  }
